vi "Pick&Place_ladder_shih_v11_MPTv2.vi"() -> ()   [LabVIEW 2016]
uses:
  WTF is this.ctl
  Classes/Controllers/I-O/Copy of NI-DAQ Folder/NI-DAQ.lvclass
  D:/INTT/V1/Classes/Controllers/I-O/Copy of I-O Folder/I-O.lvclass
  Classes/Controllers/Dispenser/Copy of Ultimus V2 Folder/Ultimus V2.lvclass
  <vilib>/Analysis/coordinate.llb/2D Cartesian Coordinate Rotation (Scalar).vi
  <vilib>/Utility/file.llb/Read Delimited Spreadsheet (DBL).vi
  <vilib>/Utility/file.llb/Write Delimited Spreadsheet (DBL).vi
  Classes/Controllers/Motion/Copy of Motion Folder/Motion.lvclass
  Classes/Controllers/Camera/Copy of Controller Folder/Controller.lvclass
  <vilib>/Analysis/NI_AALPro.lvlib
  Classes/Controllers/I-O/Copy of I-O Folder/I-O.lvclass
panel:
  out "output array":dbl[](array[numeric])
  in  "Glue hehight":dbl=1.3
  out "file indicator":dbl[][](array[numeric])
  out "?":dbl[](array[numeric]) format="%#_8g"
  in  "offset":dbl[](array[numeric])=[0.0, 0.0, 0.0, 0.0] format="%#_8g"
  out "HDI center positions":dbl[][](array[numeric]) format="%#_8g"
  out "HDI center positions":dbl[][](array[numeric])=[[459.92445114002015, 980.2358762511564, 78.77350133595746, 0.0015214873297426886]] format="%#_8g"
  out "CT sum up":dbl[](array[numeric])
  in  "txt switch":bool
  in  "MPT offset":dbl[][](array[numeric])=[[0.0, 0.0, 0.0, 0.0], [0.0, 0.0, 0.0, 0.0]] format="%#_8g"
  out "CT HPoS":dbl[][](array[numeric]) format="%#_8g"
  out "chip distance by OGP":dbl format="%#_8g"
  out "displacement":dbl[](array[numeric])
  out "gantry position test":dbl[](array[numeric])
  out "gantry target position":dbl[](array[numeric])
  out "chip distance by gantry":dbl format="%#_8g"
  out "after SL":dbl[](array[numeric]) format="%#_8g"
  out "after SR":dbl[](array[numeric]) format="%#_8g"
  out "after NL":dbl[](array[numeric]) format="%#_8g"
  out "S chip":dbl[](array[numeric]) format="%#_8g"
  out "N chip":dbl[](array[numeric]) format="%#_8g"
  in  "?":path=path "C:/Users/PAGANIS/Desktop/shih cheng wei/OGP/test1-2.txt"
  out "bless from OGP !!! Center of  stave":dbl[](array[numeric])
  out "bless from OGP !! measured stave size":dbl[](array[numeric])
  in  "Bless from OGP":bool
  out "FROM Detail !!! Center of module on stave":dbl[](array[numeric])
  out "FROM Detail !! measured stave size":dbl[](array[numeric])
  in  "Align Stave in detail":bool
  in  "Uttimus presssure":i64=10
  out "Status":bool
  out "measured HDI top-left position":dbl[][](array[numeric])
  in  "HDI vacuum channel":i32=18
  in  "vacuum":bool=TRUE
  in  "HDI vacuum":bool
  out "measured stave size":dbl[](array[numeric])
  out "Stave mark":dbl[][](array[numeric])
  out "Center of module on stave":dbl[](array[numeric])
  out "Measured HDI size":dbl[][](array[numeric])
  out "MPT positions on stave":T1[][](array[typedef])
  in  "Default Stave dimension":dbl[](array[numeric])=[34.0, 472.0, -0.335295, -0.000320234]
  in  "Default Stave upper left mark":dbl[](array[numeric])=[584.376, 675.576, 70.9882, 0.000840064]
  out "Needle parking position":dbl[](array[numeric])
  in  "Uppler / Lower Stave":bool=TRUE
  out "Gantry current position":dbl[](array[numeric])
  in  "READ Position":bool
  in  "Needle Height Compenstation\n(glue gap)":dbl=0.33
  in  "Needle Alignment":bool
  in  "Parking position":dbl[](array[numeric])=[625.0, 625.0, 0.0, 0.01]
  in  "GOTO":bool
  in  "Default Pickup Tool Position":dbl[][](array[numeric])=[[152.226, 682.729, 36.8129, -0.0151898], [700.0, 800.0, 20.0, 0.01]]
  in  "deposit glue module":i32=1
  in  "Default HDI alignment \nmark position":dbl[](array[numeric])=[448.322, 976.582, 74.9872, 0.000191129]
  in  "Default HDI size":dbl[](array[numeric])=[24.2437, 231.446, -0.099339, 0.000191129]
  out "# of tasks excuted":i32
  out "PickupTool \nCenterPosition":dbl[](array[numeric]) format="%#_8g"
  in  "Inititalize":bool
  in  "Pick and place":bool
  in  "Deposit Glue":bool
  in  "Measure Pickup Tools":bool
  in  "Align Stave":bool
  out "default module position on stave":dbl[][](array[numeric])
  in  "Stop":bool
  in  "Measure HDI":bool
  # "Ladder Assembly"
  # "To switch the north/south\ntxt file \nswitch \noffset\nmodule pick up tool\nmodule direction"
  # "upper : north \nlower : south"
  # "Sensor 0.32 -> 200 micron glue thickness\nChips 0.37-> 140 micron glue thickness"
  # "Upper\nmodule"
  # "Lower\nmodule"
  # "ACTIONS"
  # "theta had *-1"
  # "Pick up tool and needle"
  # "Module infomation"
  # "Pick and Place"
  # "after assembly"
  # "CT"
  # "+"
  # "+"
  # "="
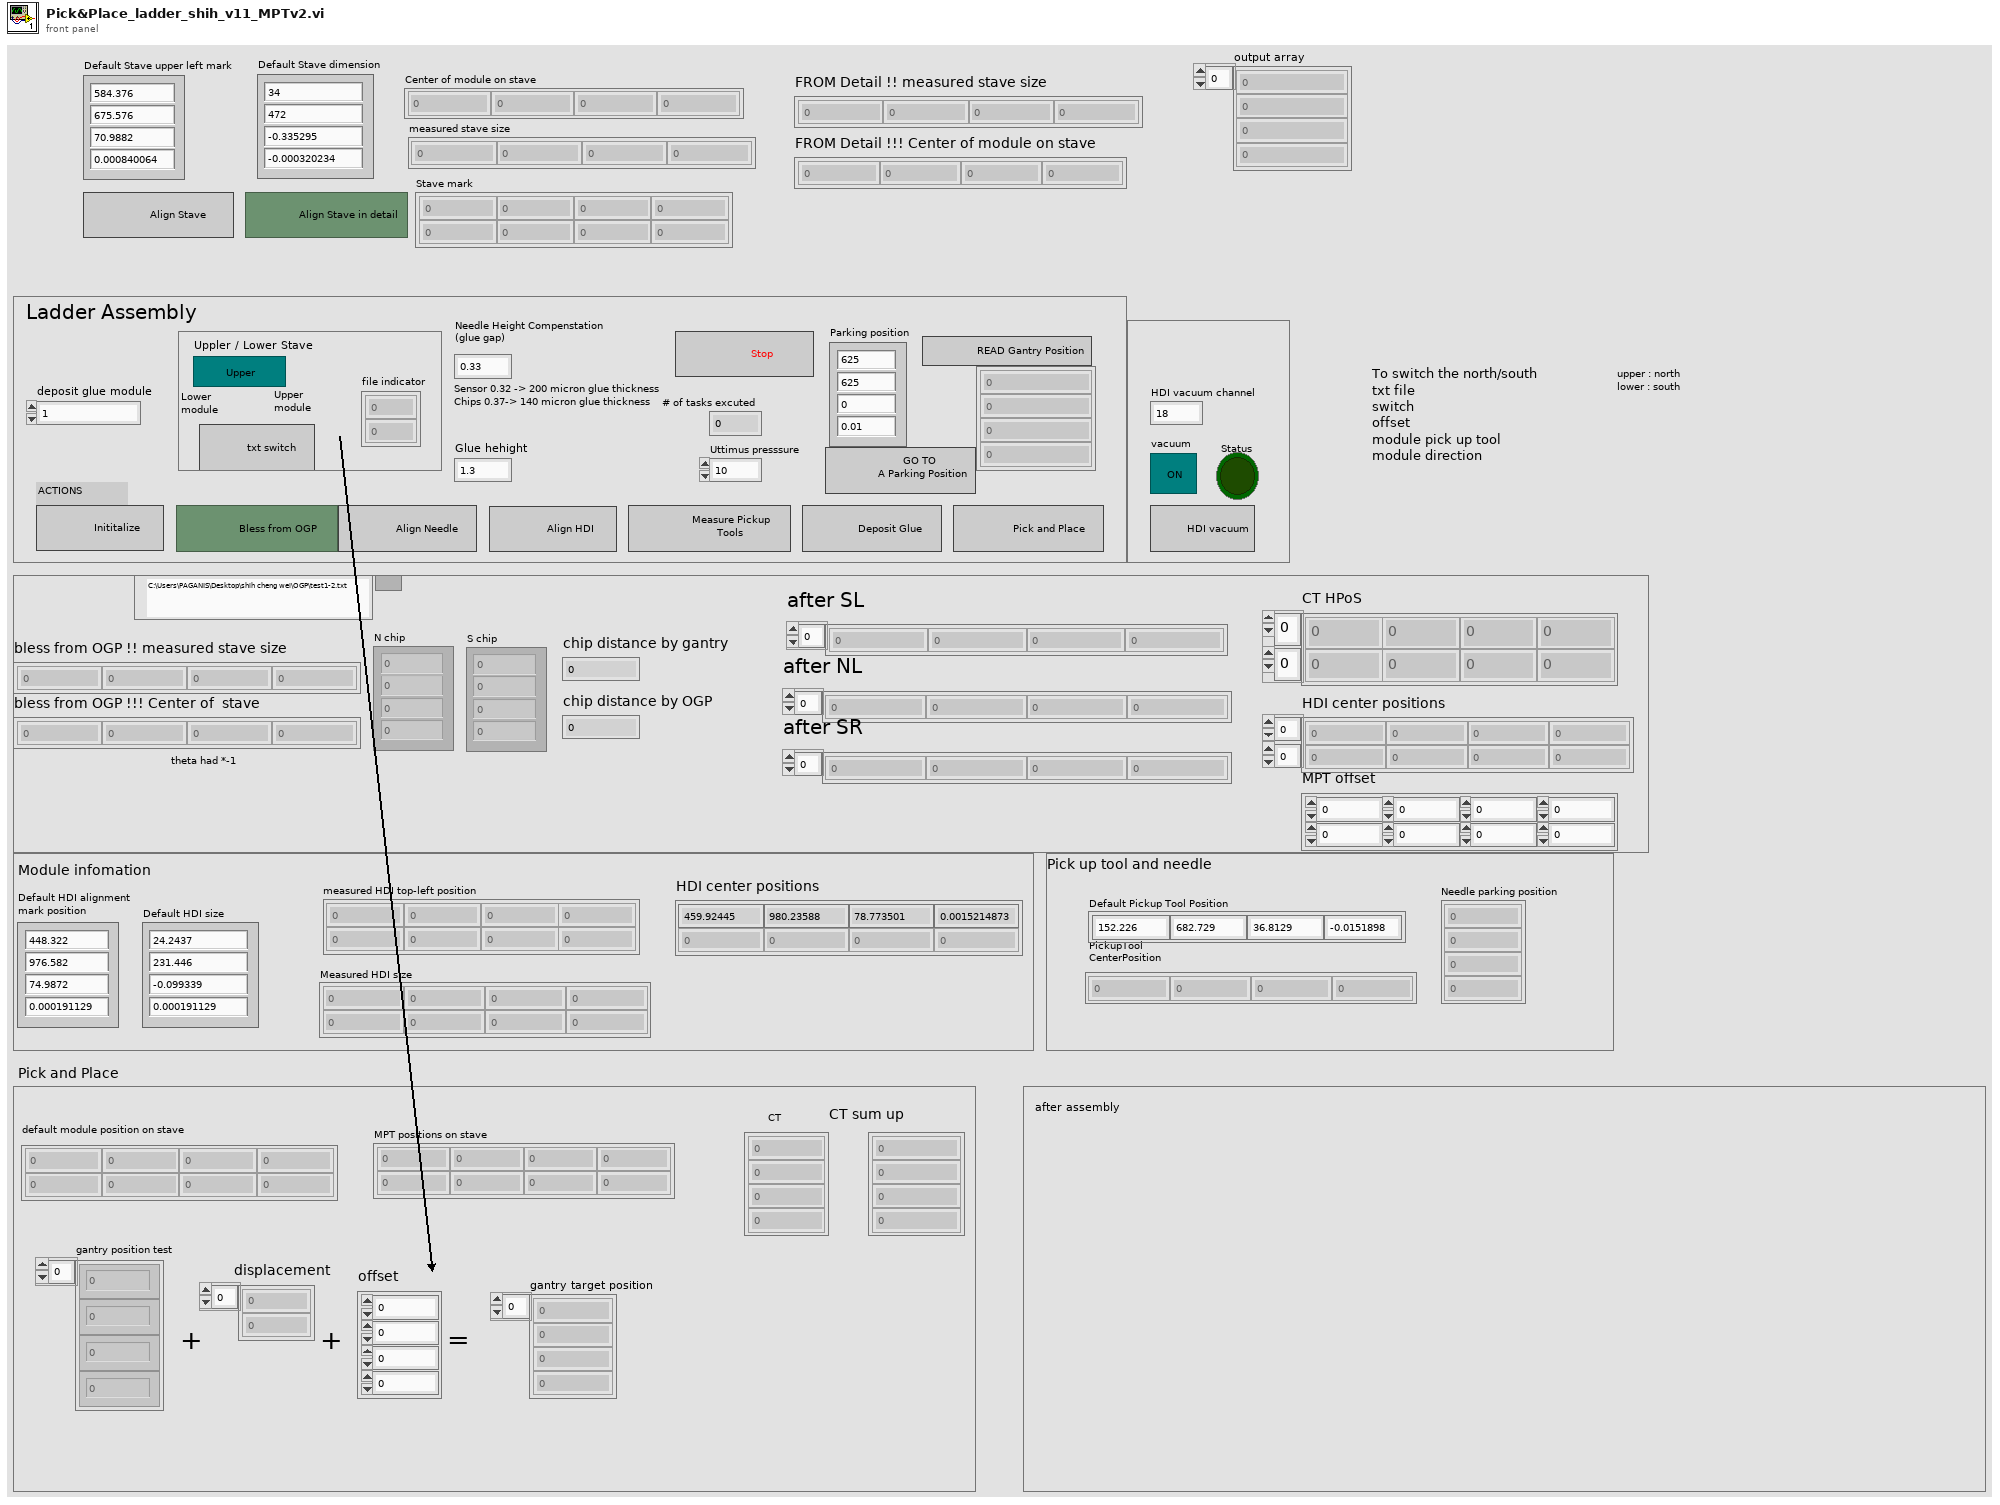
[diagram p1: front panel]
types:
  T1 = typedef "WTF is this.ctl" = dbl
  T2 = typedef "Controller.lvclass/Controllers.ctl" = cluster{"Copy of Motion.lvclass":refnum<class "Motion.lvclass">, "Copy of I-O.lvclass":refnum<class "I-O.lvclass">, "Copy of Dispenser.lvclass":refnum<class "Dispenser.lvclass">}
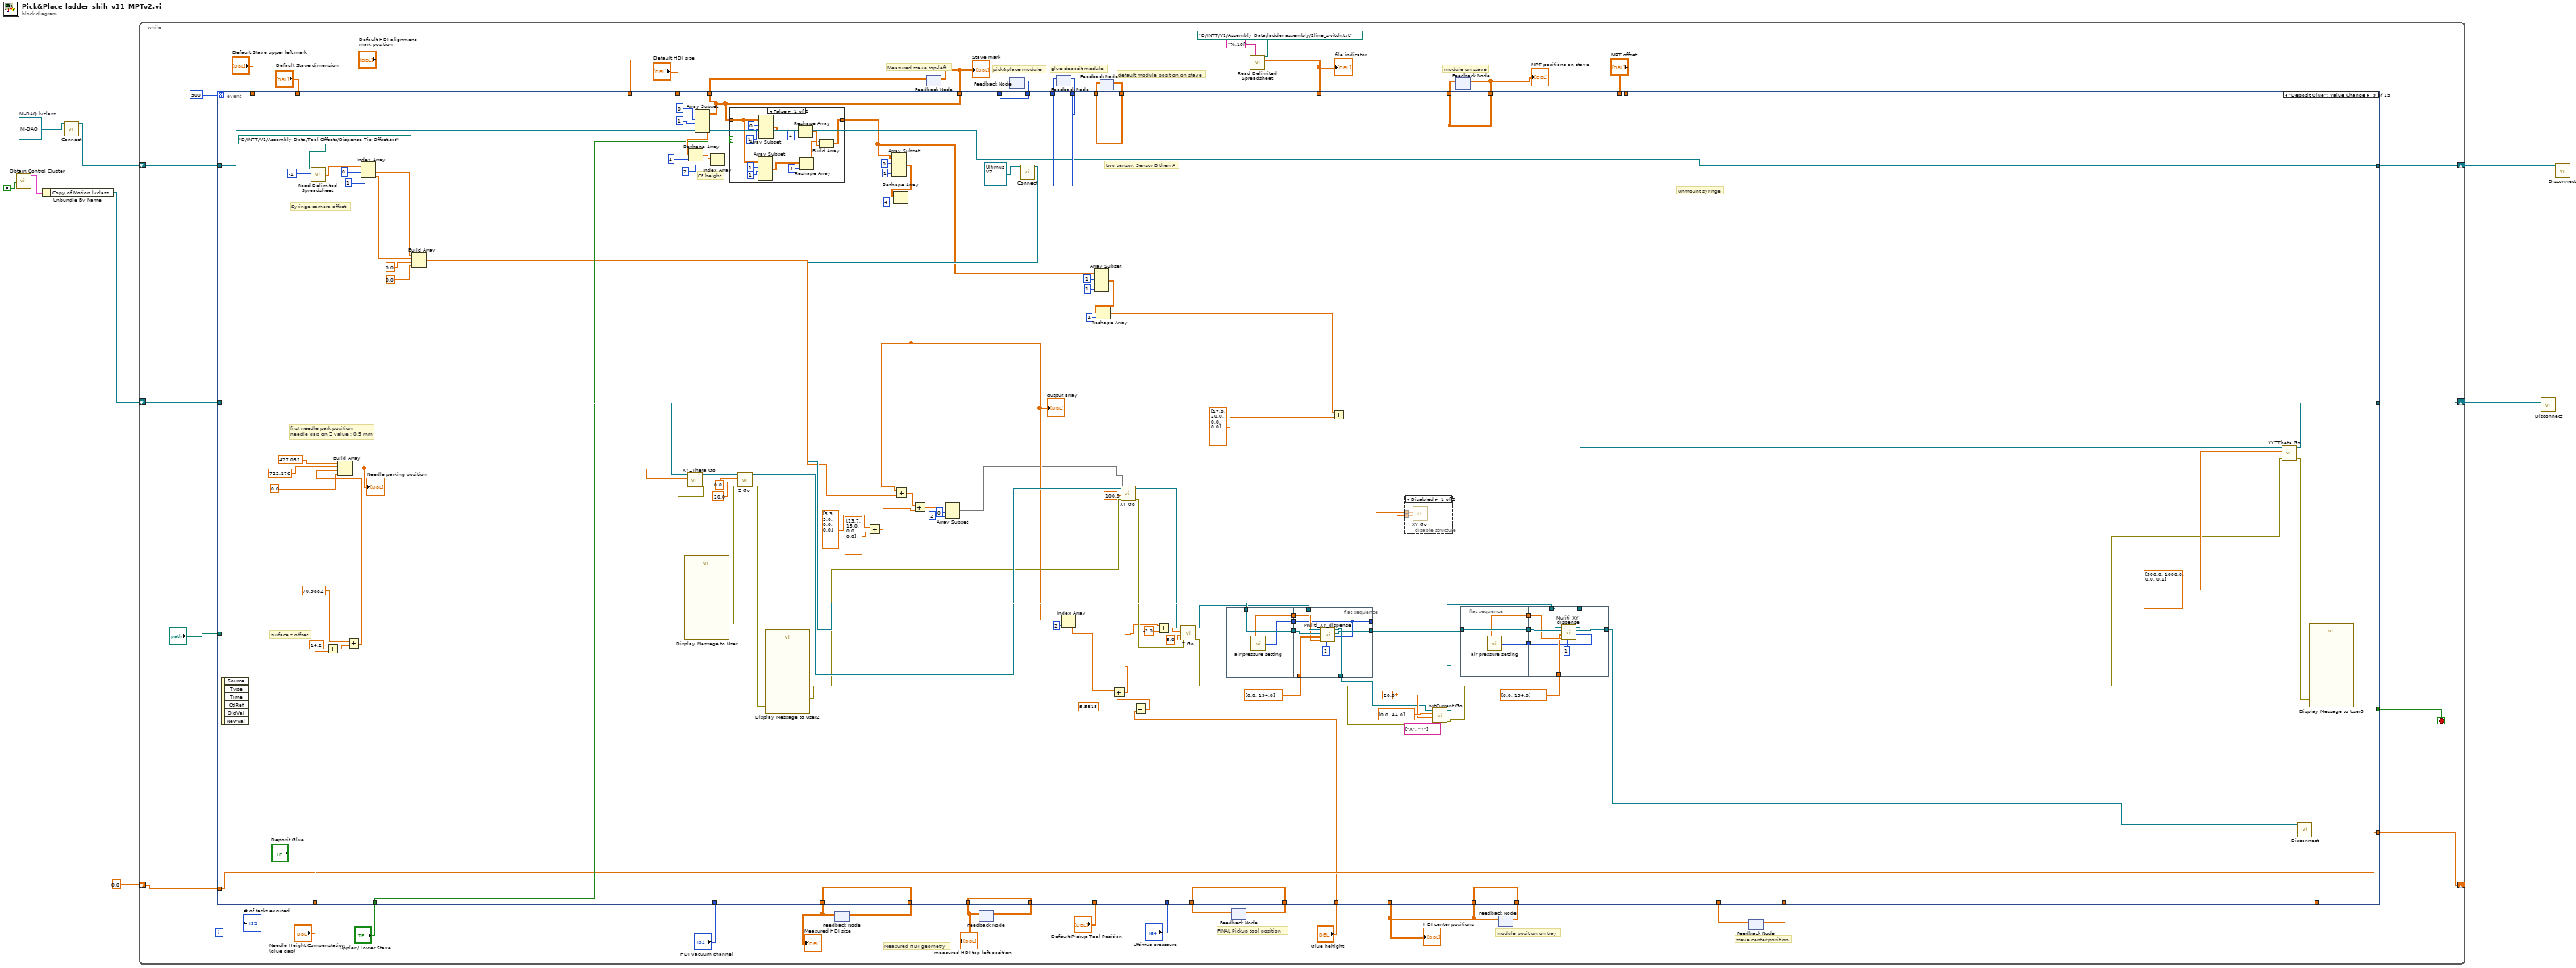
[diagram p0: block diagram]
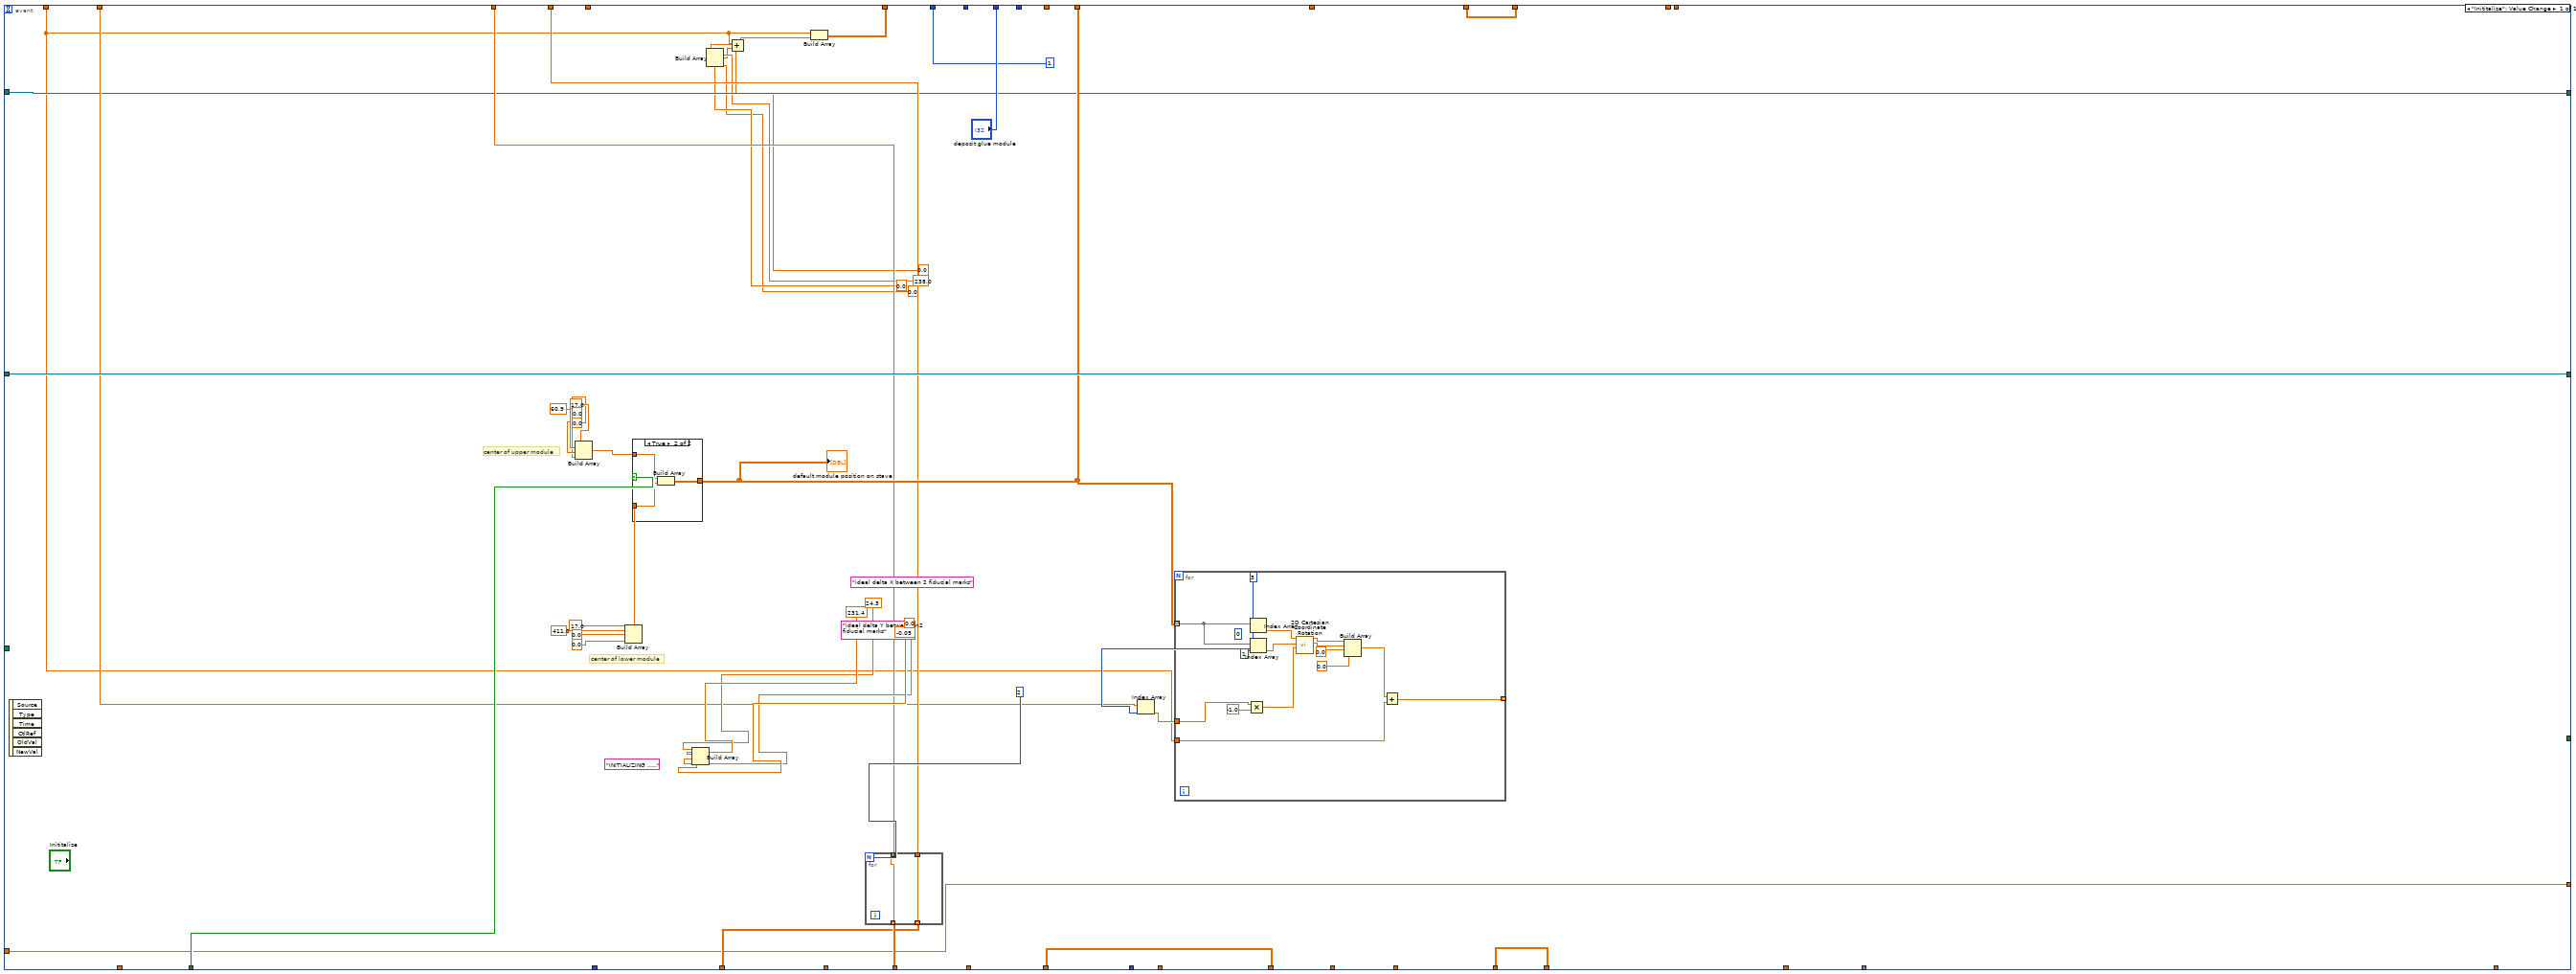
[diagram p2: hidden frame]
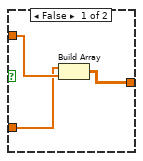
[diagram p3: hidden frame]
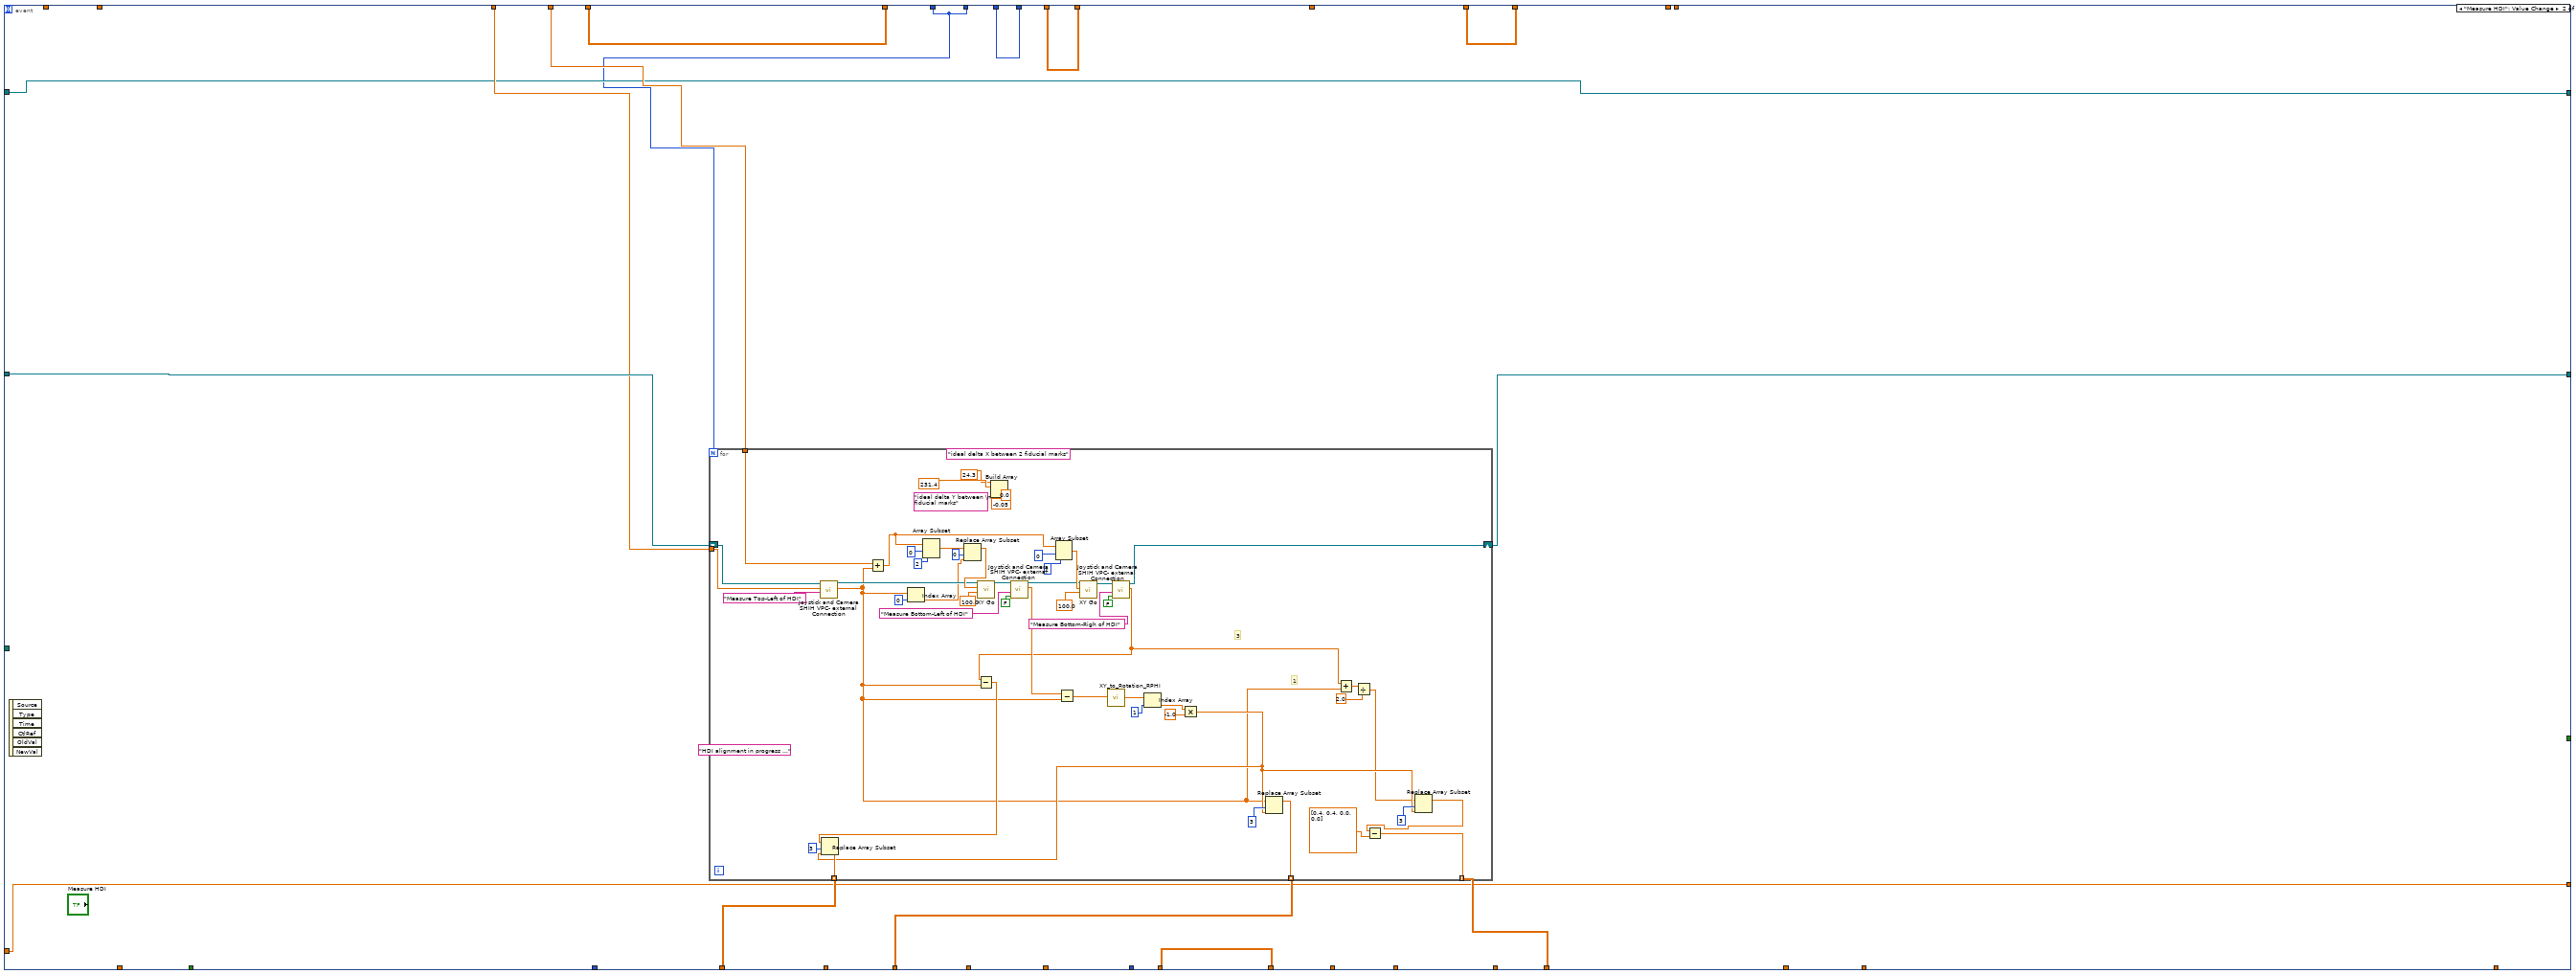
[diagram p4: hidden frame]
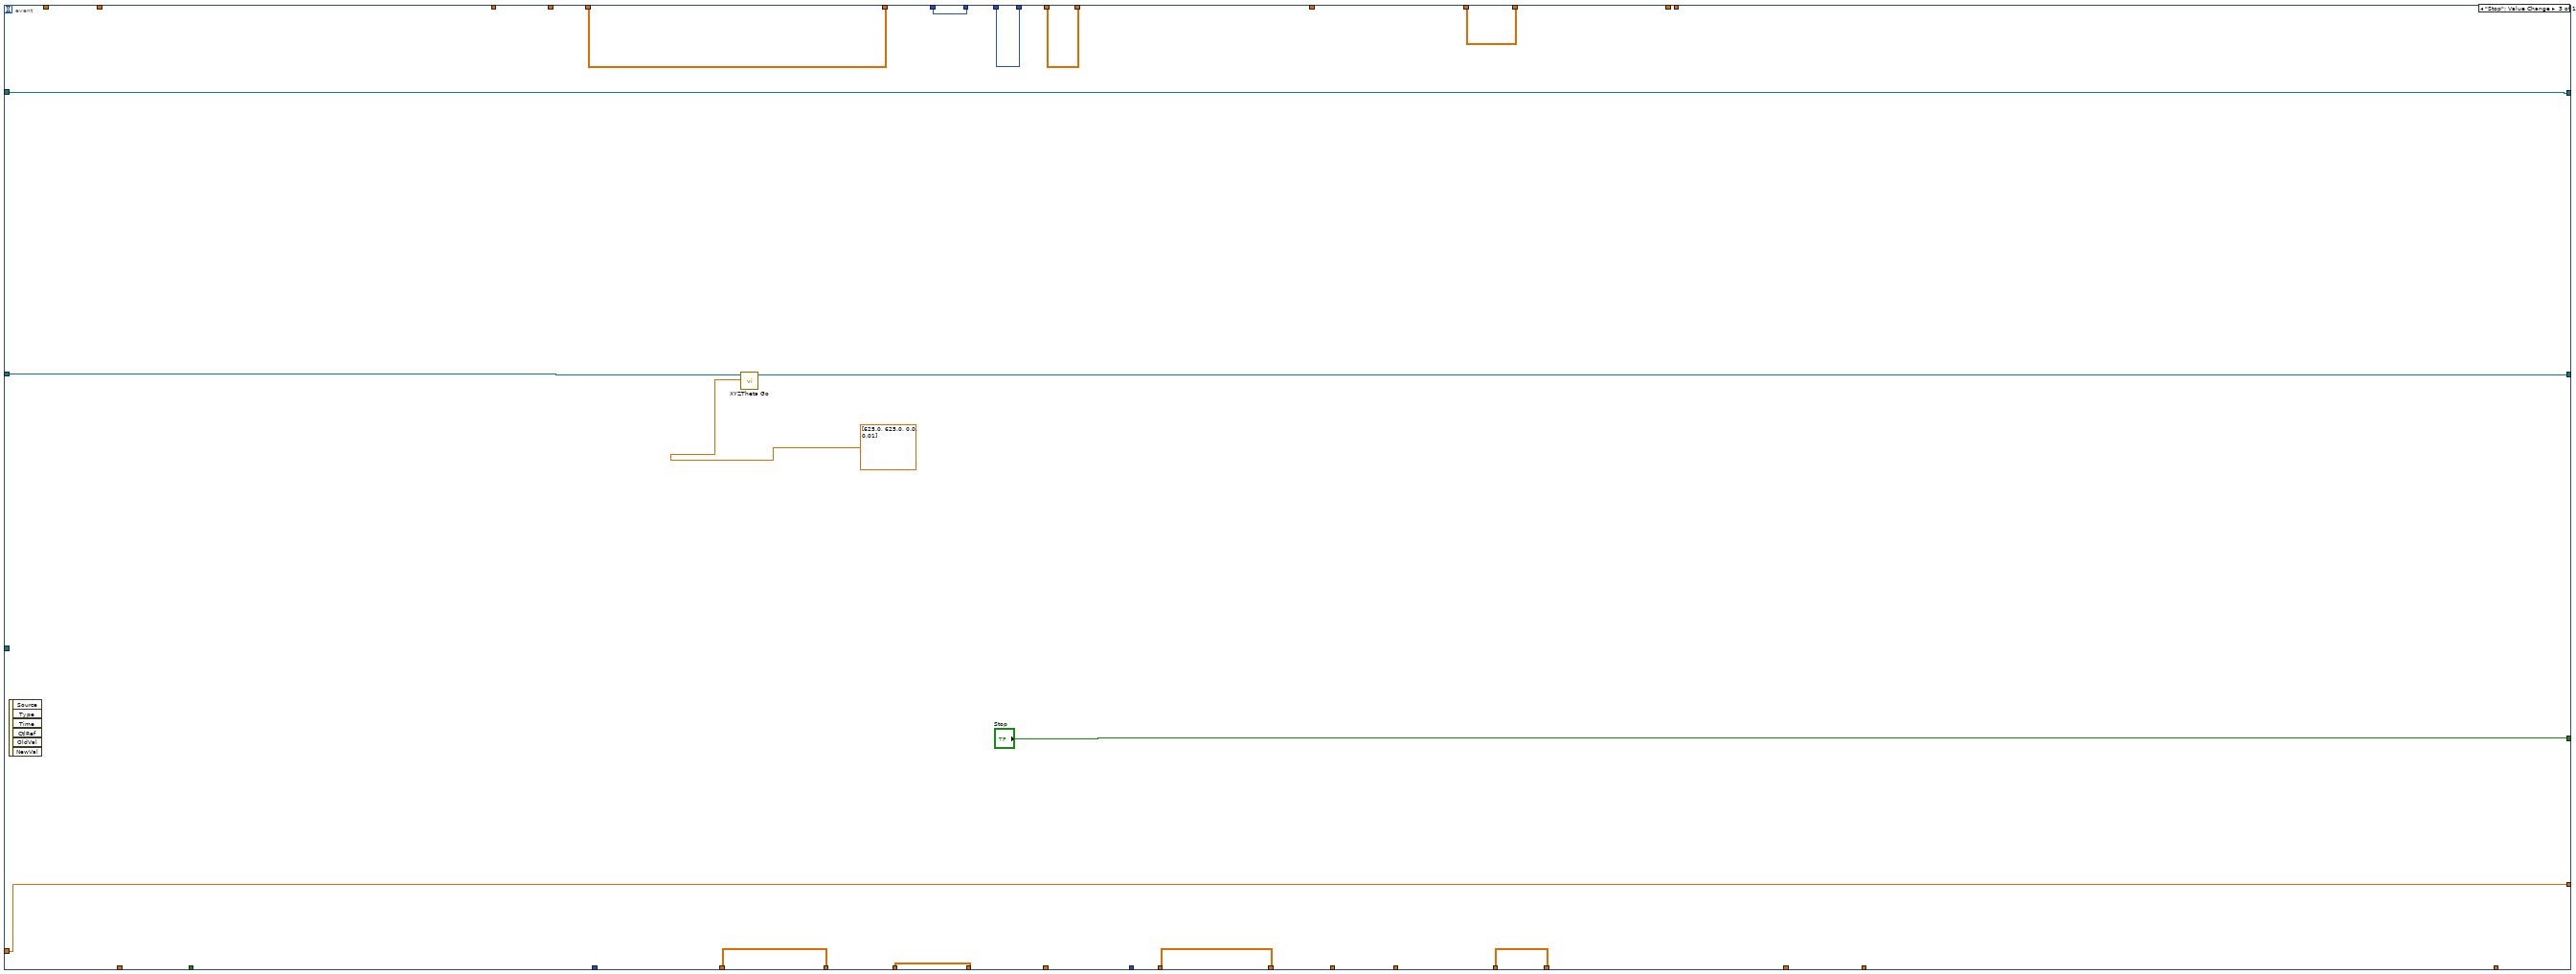
[diagram p5: hidden frame]
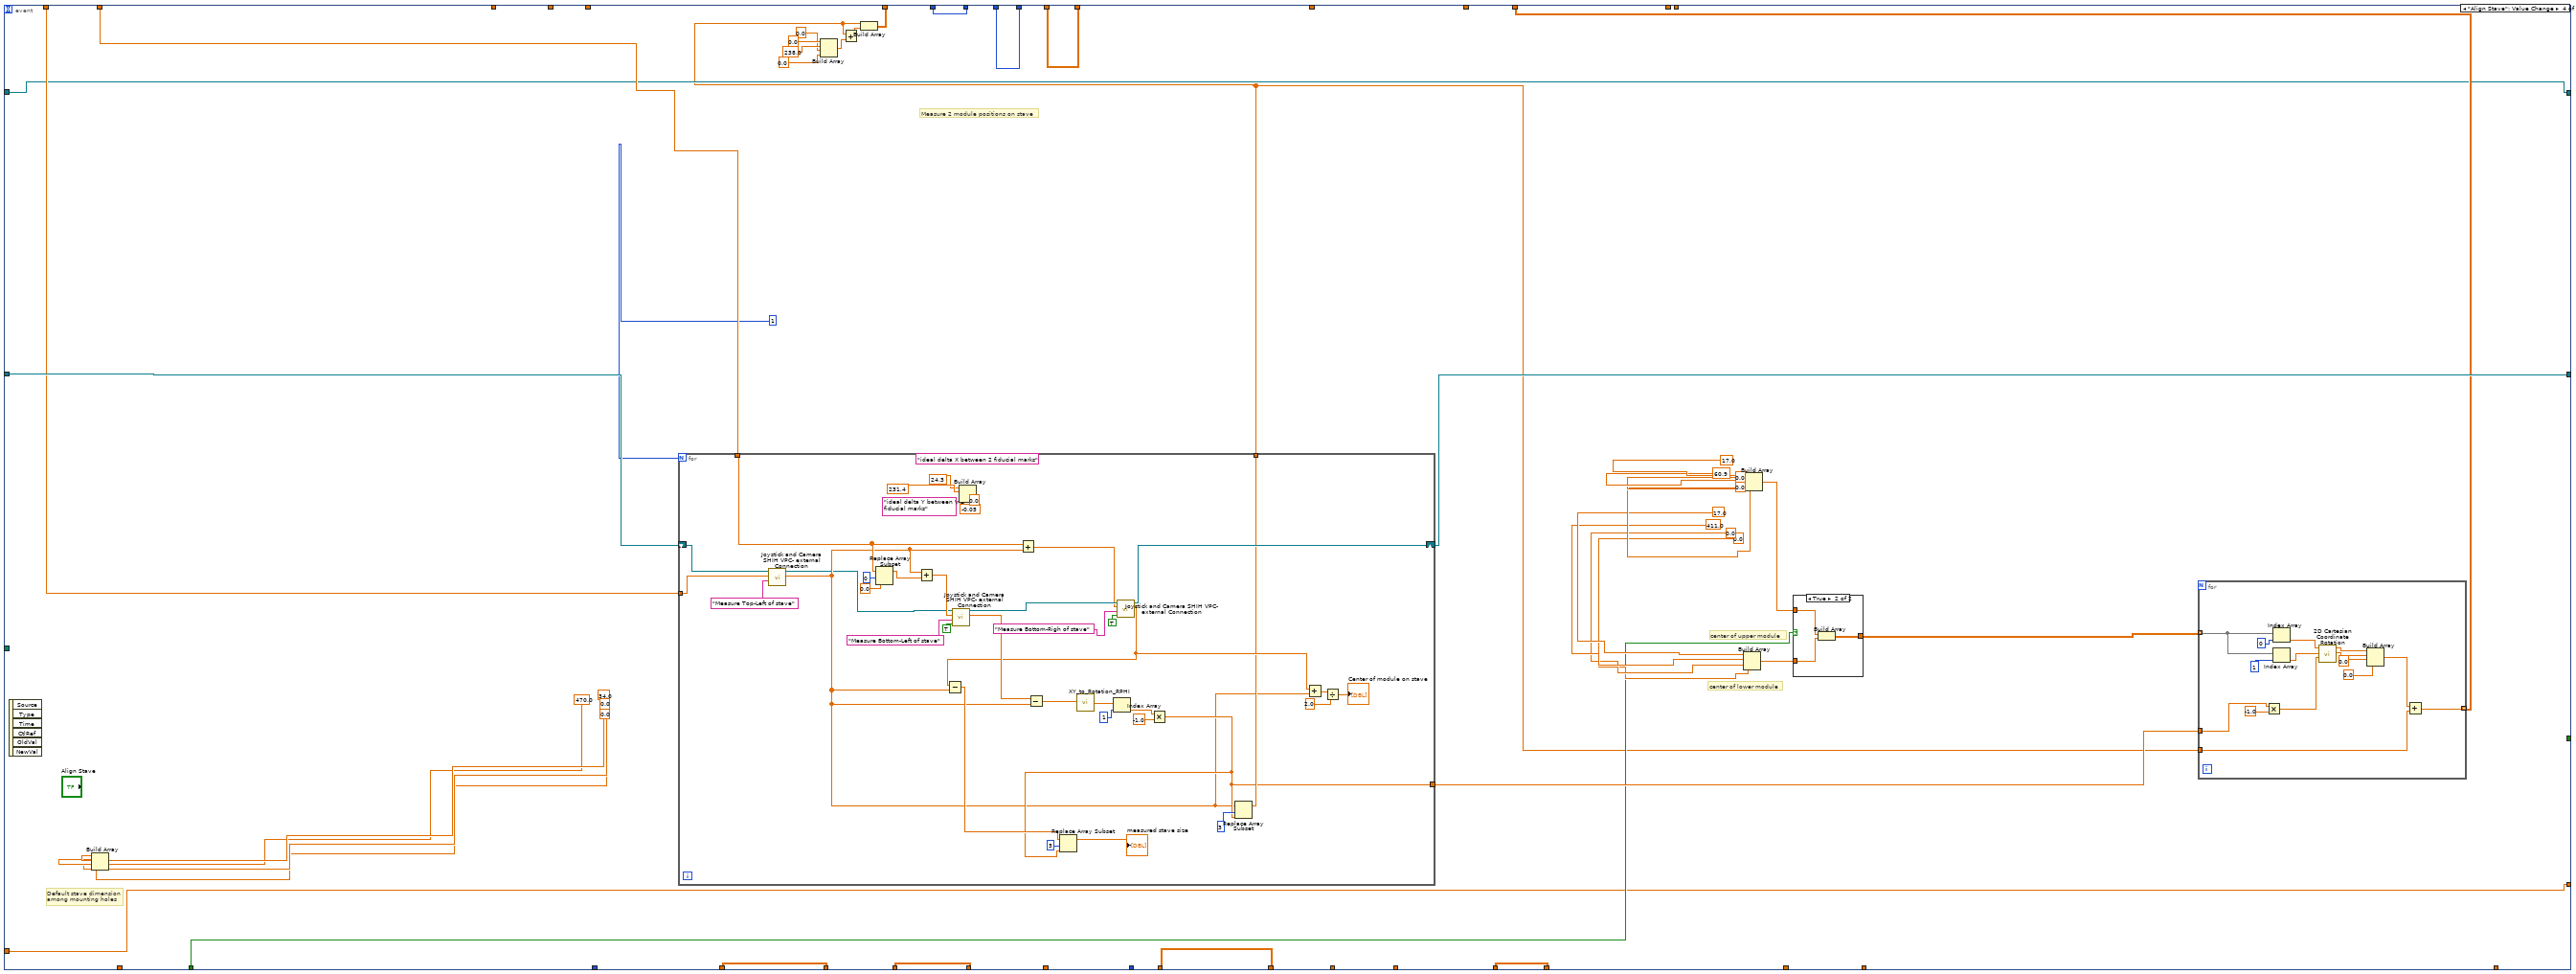
[diagram p6: hidden frame]
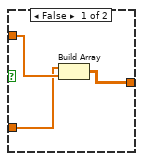
[diagram p7: hidden frame]
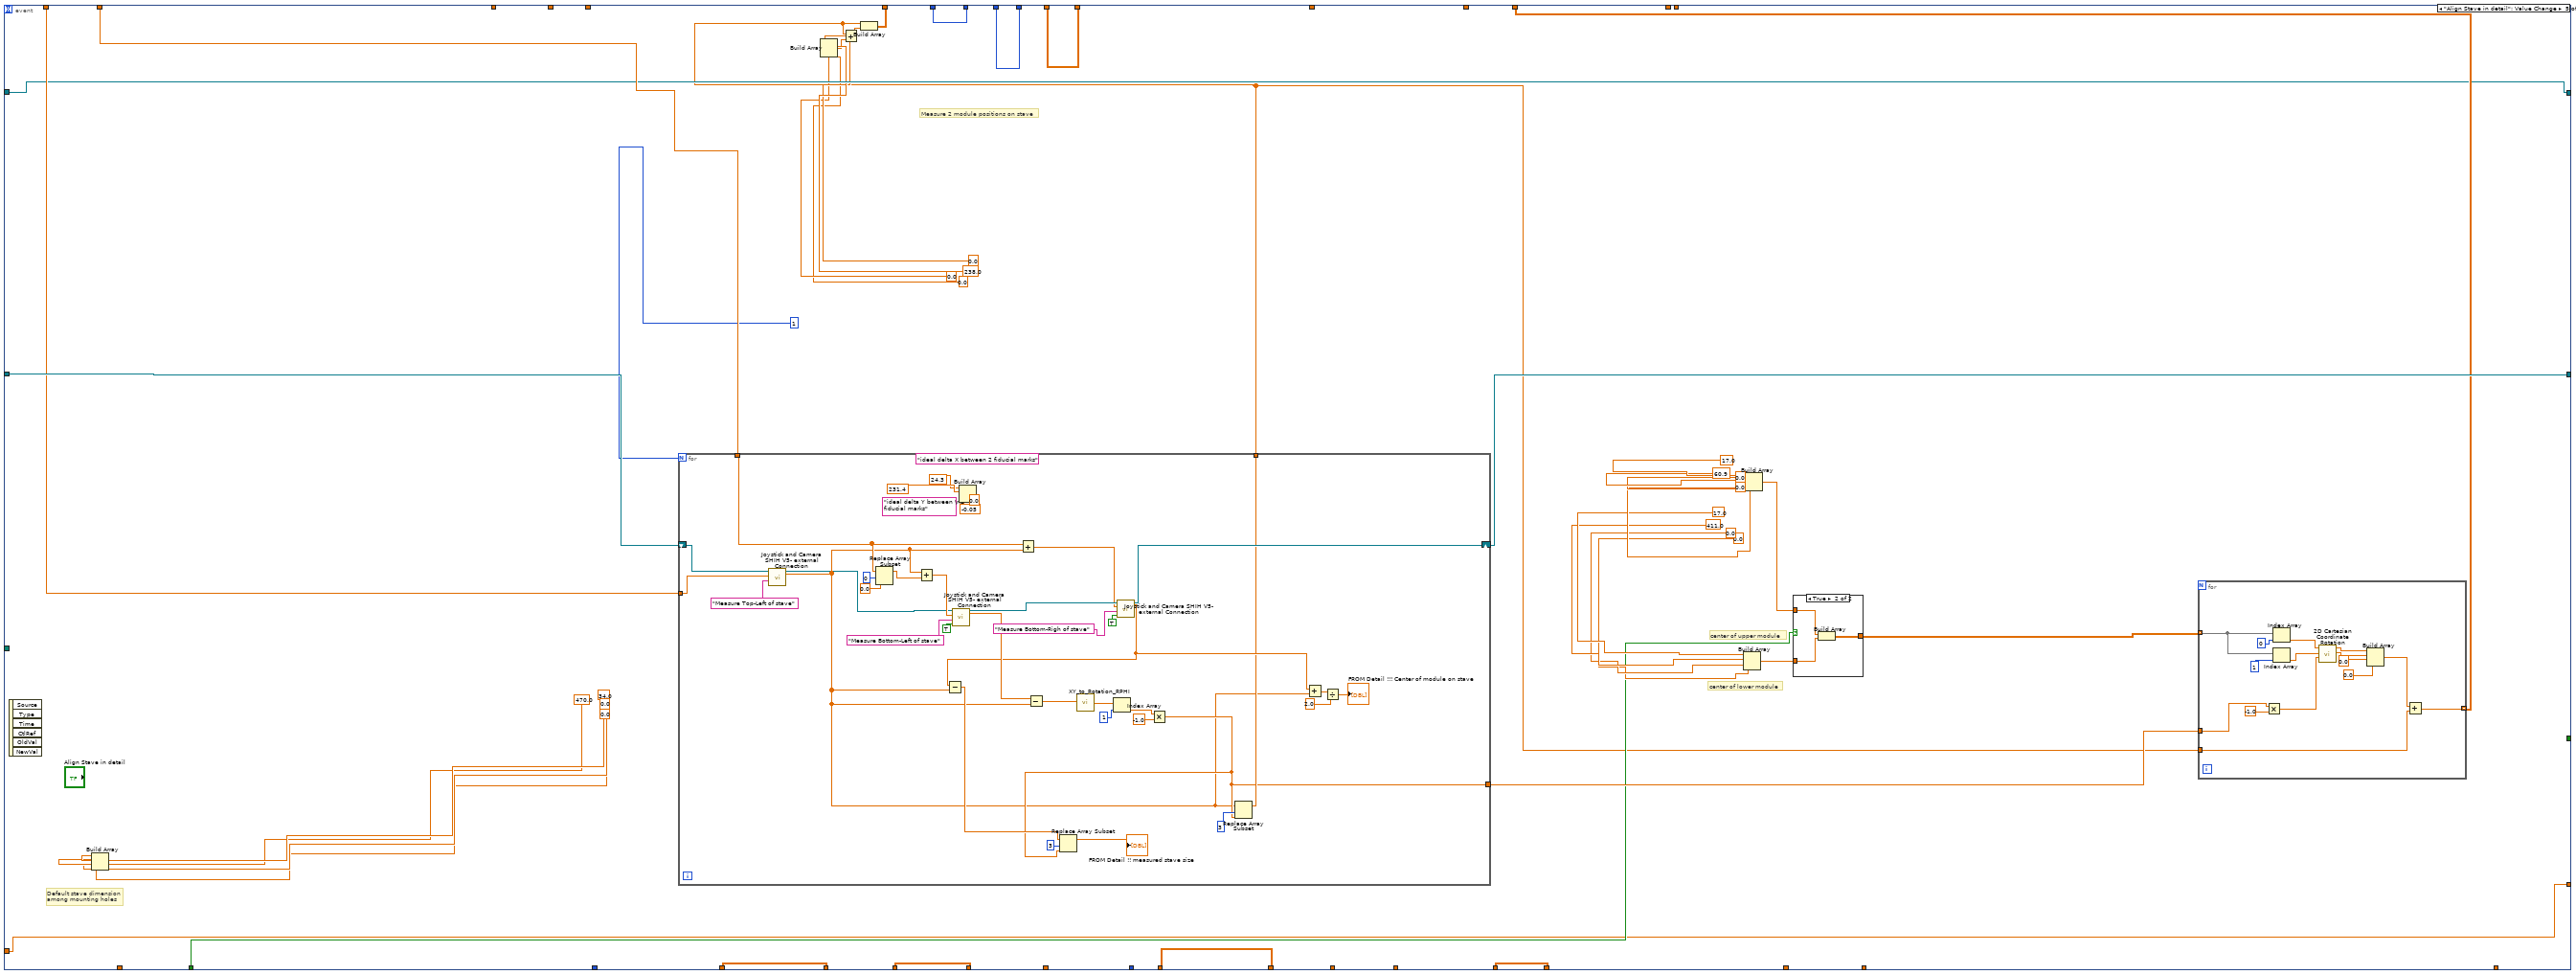
[diagram p8: hidden frame]
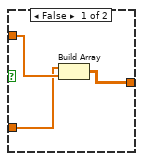
[diagram p9: hidden frame]
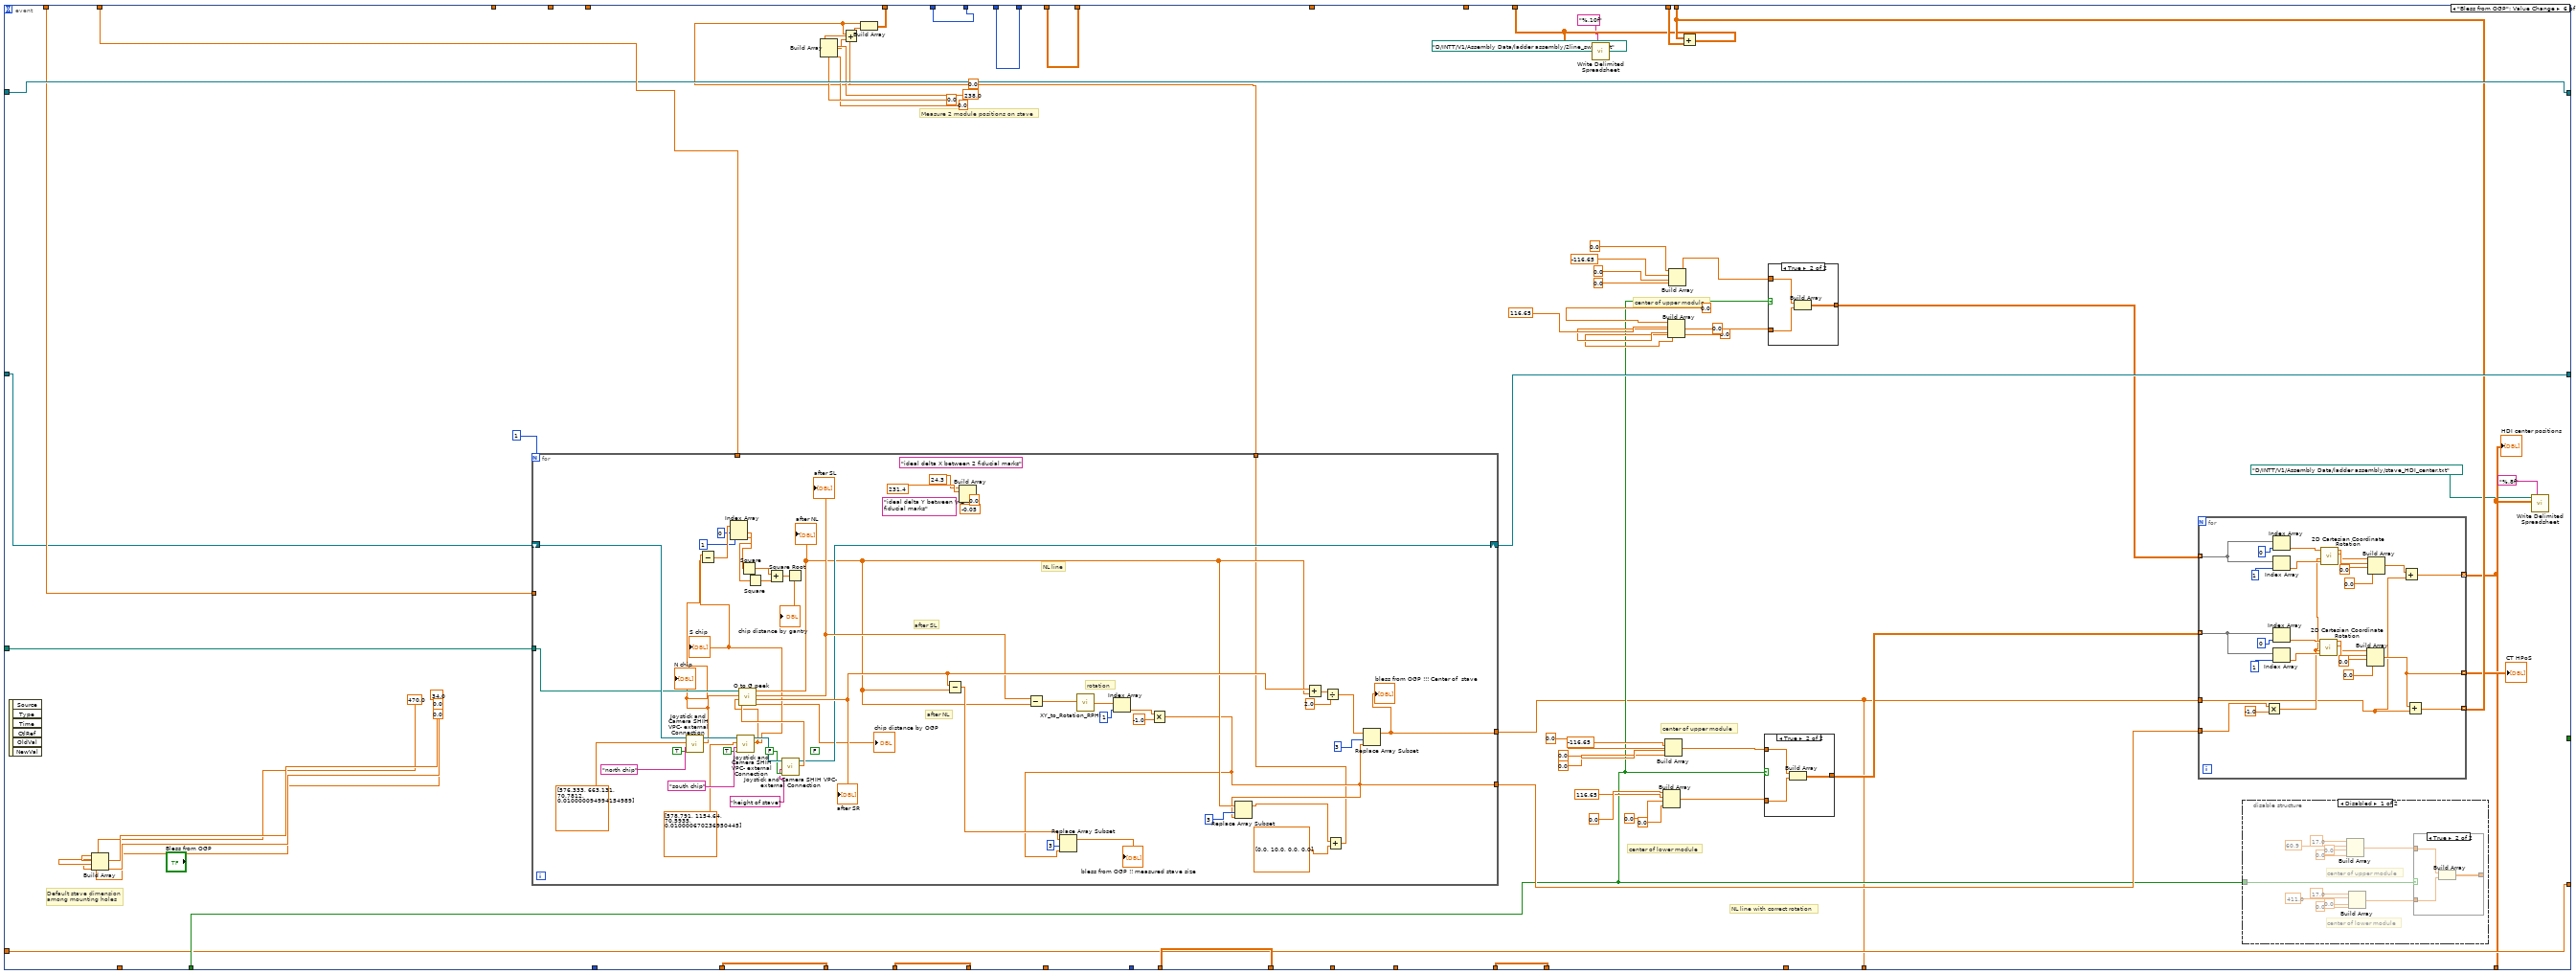
[diagram p10: hidden frame]
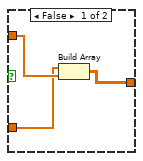
[diagram p11: hidden frame]
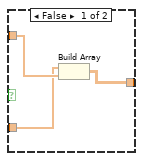
[diagram p12: hidden frame]
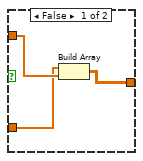
[diagram p14: hidden frame]
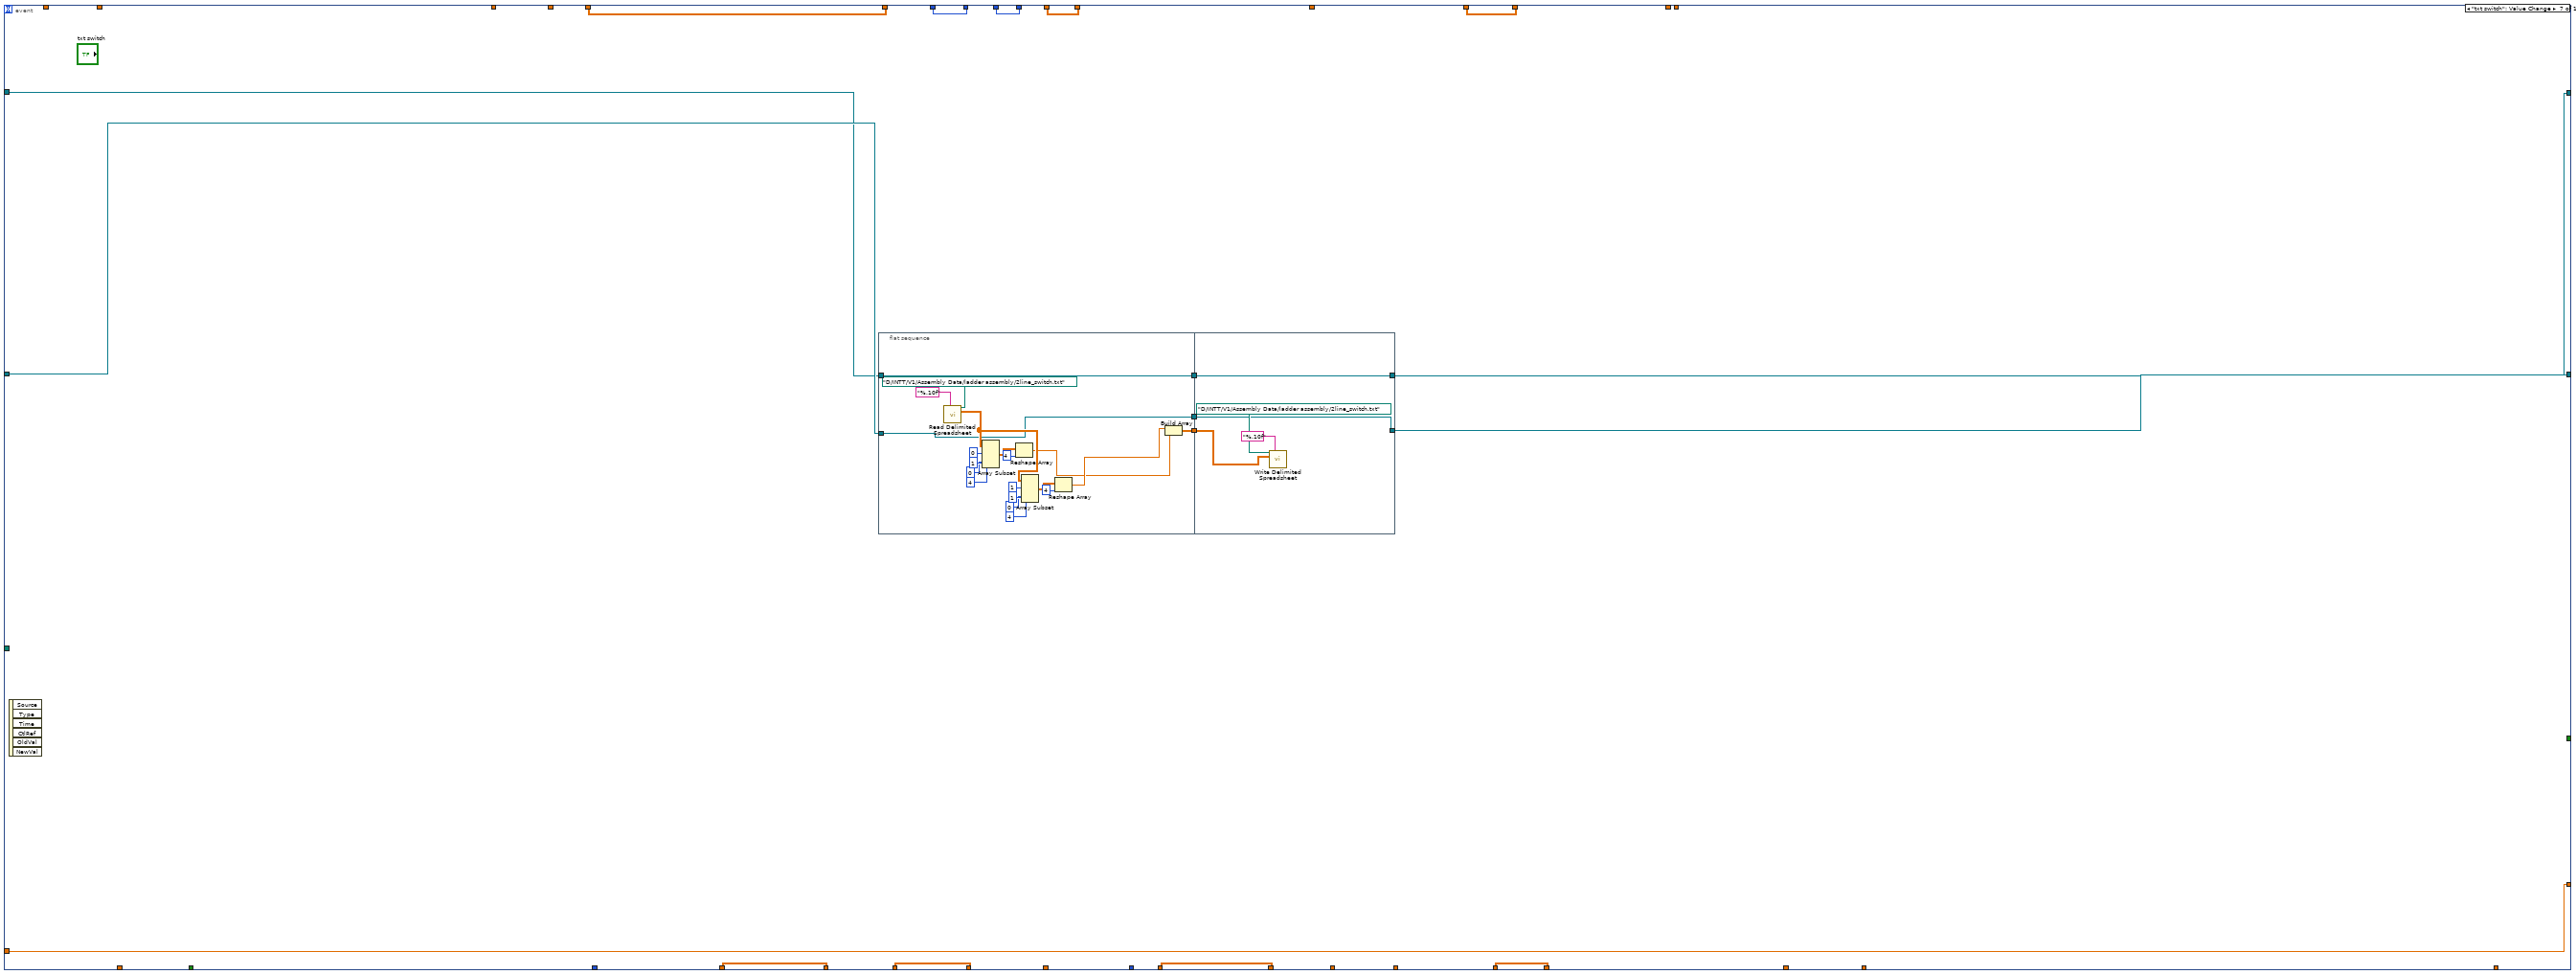
[diagram p15: hidden frame]
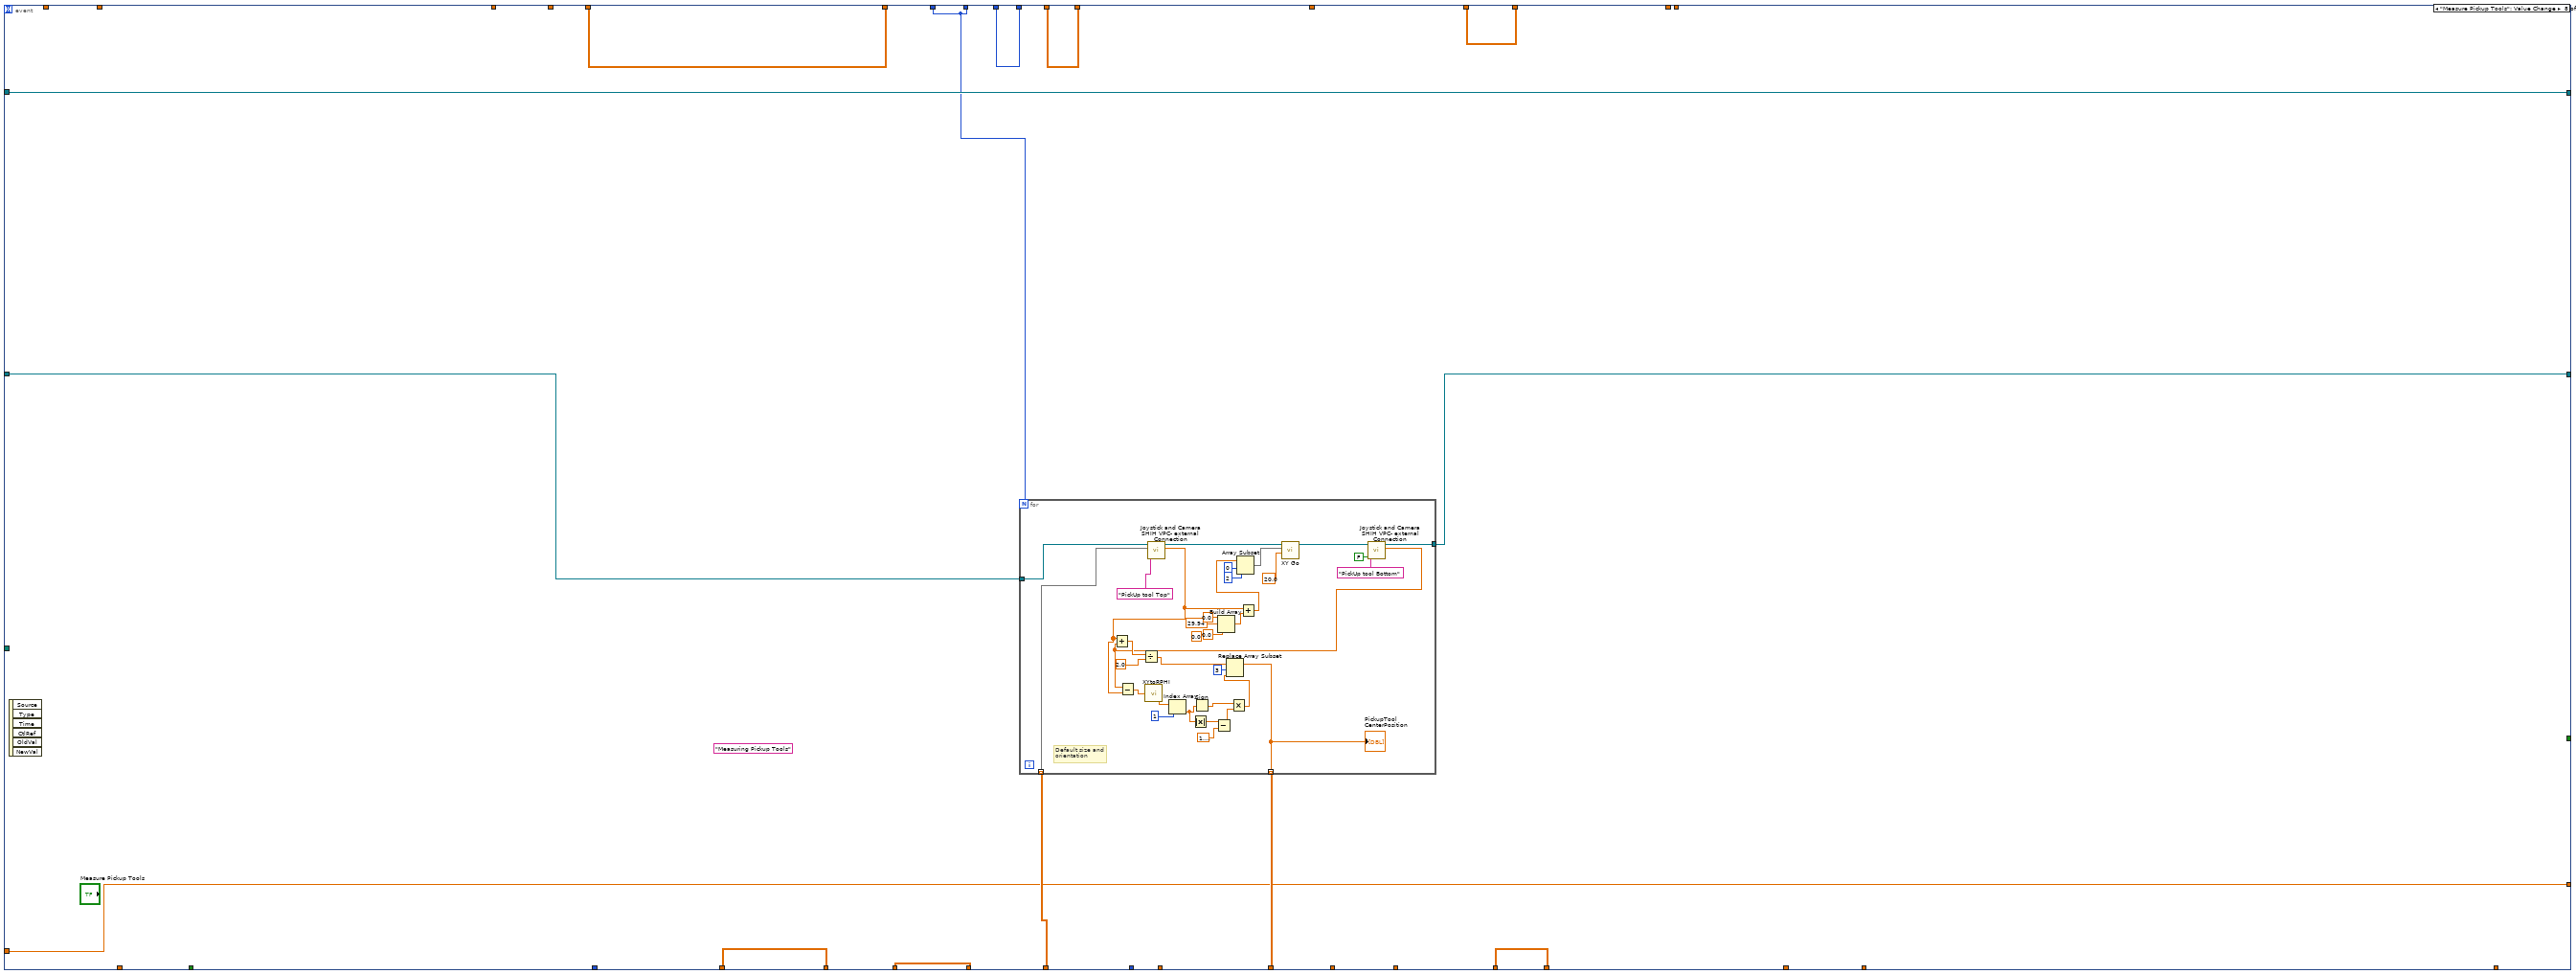
[diagram p16: hidden frame]
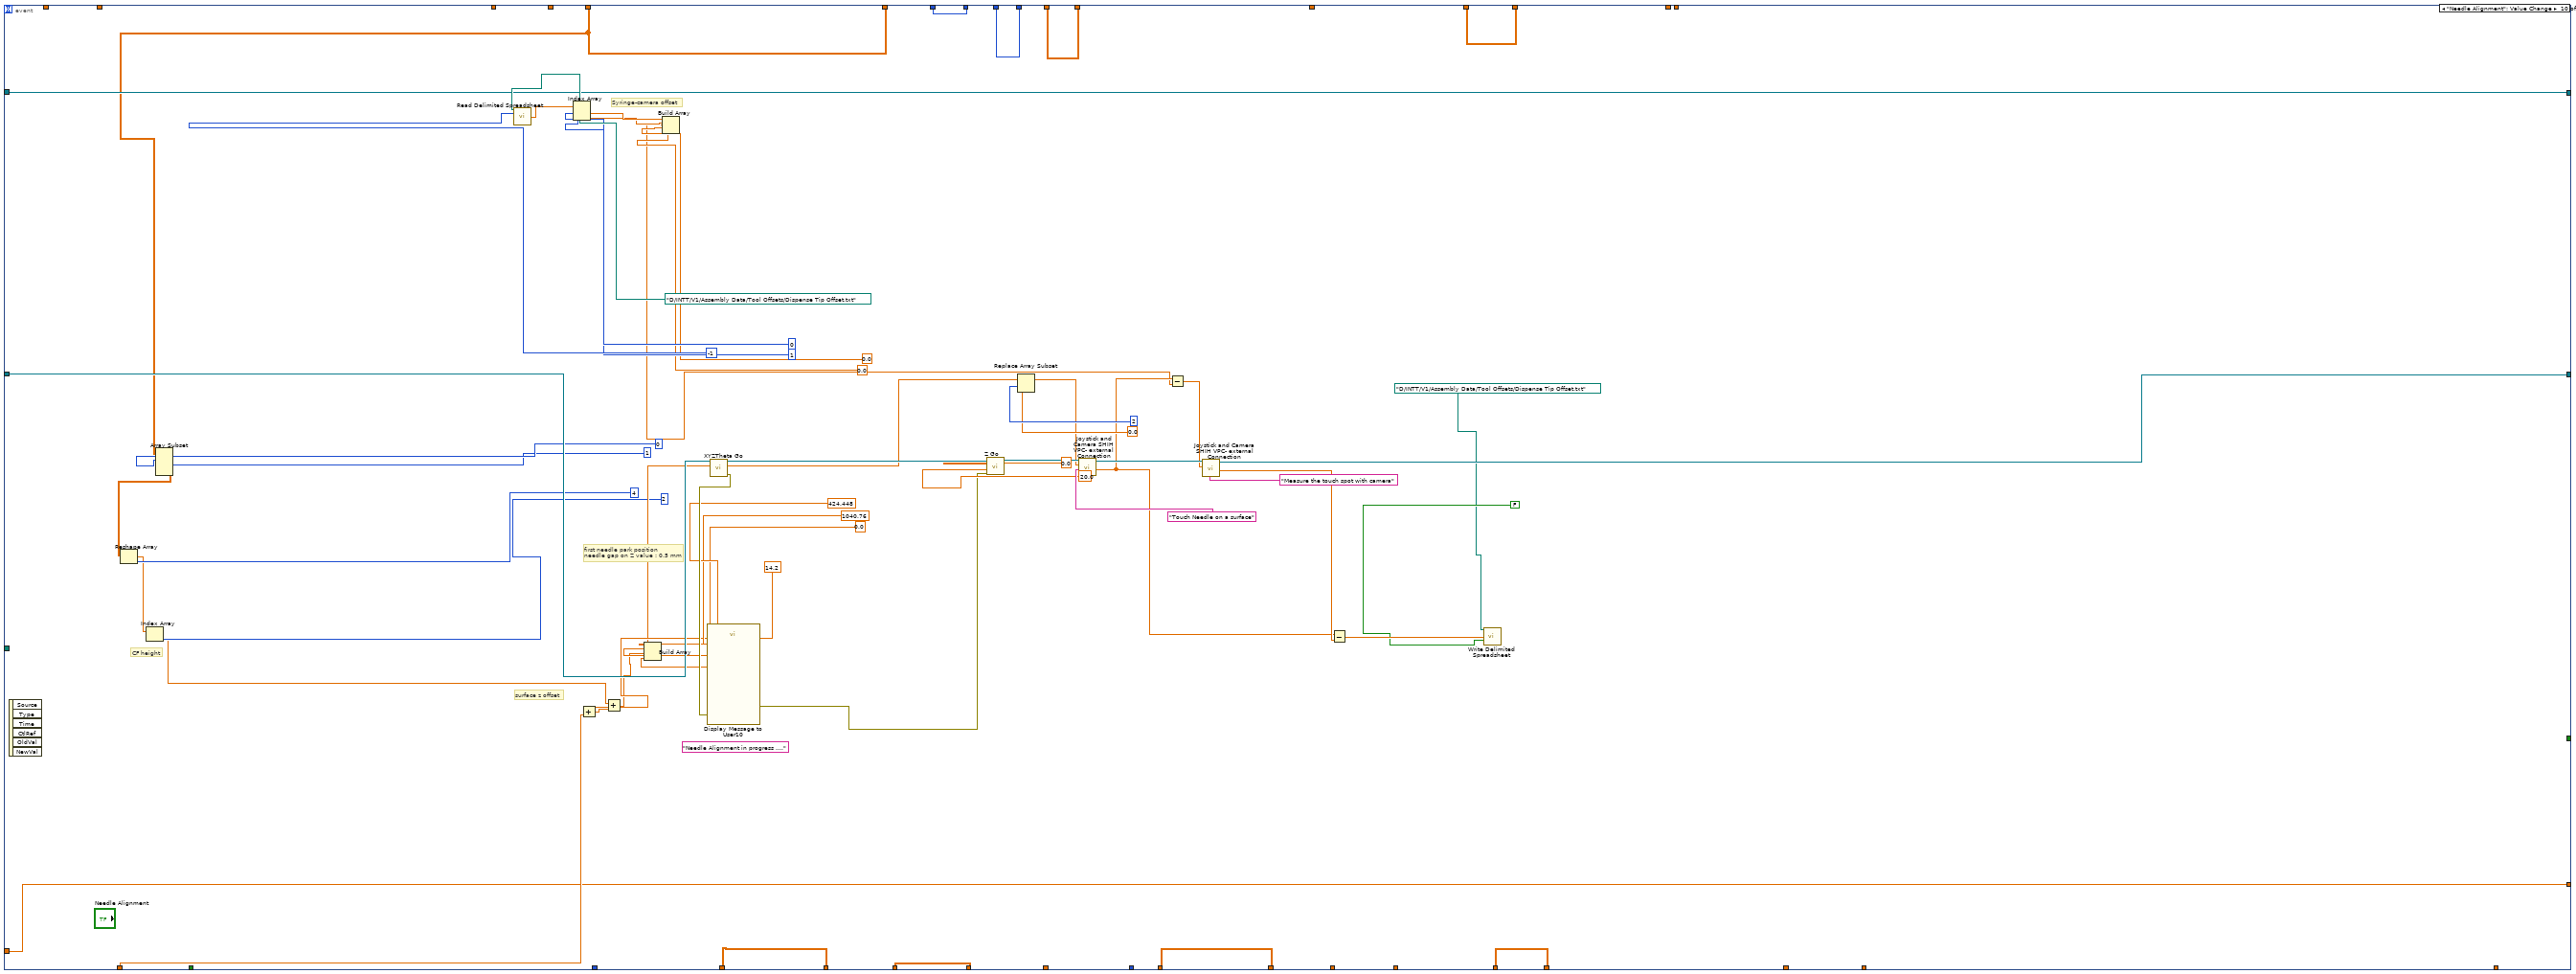
[diagram p19: hidden frame]
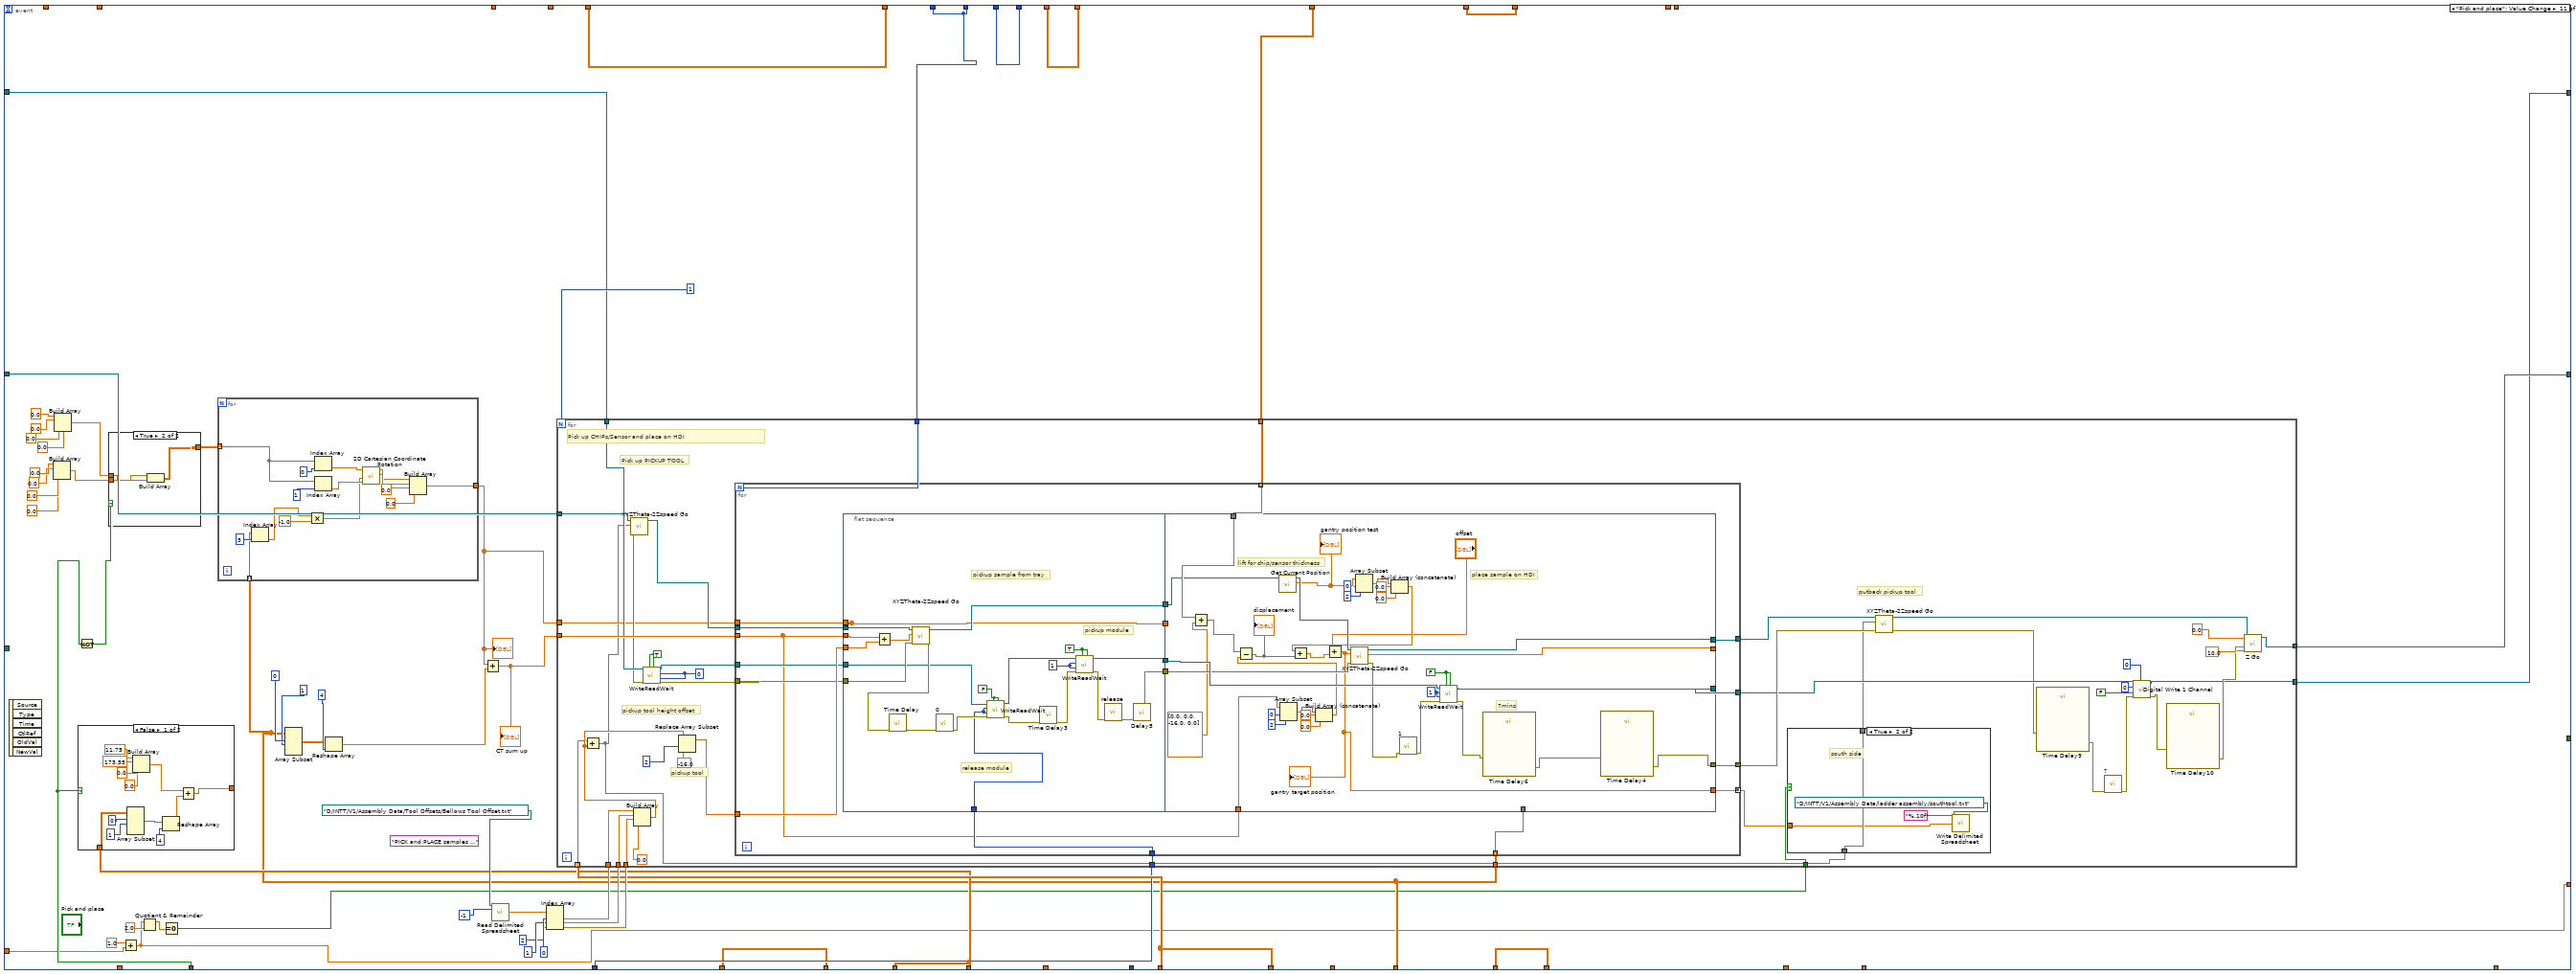
[diagram p20: hidden frame]
diagram:
  w4 = refnum<class "NI-DAQ.lvclass"> refnum  # NI-DAQ.lvclass
  n1 = call "Obtain Control Cluster.vi"("I/O"=FALSE) -> ("Control Out"=w8:T2)  [unwired: 10 in]
  n2 = Unbundle By Name(w8) -> ("Copy of Motion.lvclass"=w6:refnum<class "Motion.lvclass">)
  n3 = call-dynamic "Connect.vi"("NI-DAQ in"=w4) -> ("NI-DAQ out"=w3:refnum<class "NI-DAQ.lvclass">)  [unwired: 9 in, 1 out]
  n4 = while {
    shift-right: [w45] -> w5
    shift-left: w6 -> [w52]
    shift-right: [w25] -> w2
    shift-left: w3 -> [w29]
    shift-right: [w12] -> _
    shift-left: 0.0 -> [w13]
    i -> [w44]
    stop <- w51 stop-if-true
    # "stave center position"
    # "pick&place module"
    # "default module position on stave"
    # "FINAL Pickup tool position"
    # "glue deposit module"
    # "Measured HDI geometry"
    # "module position on tray"
    # "Measured stave top-left"
    # "module on stave"
    n5 = feedback #1() -> (w49:dbl[][])  [unwired: 1 in]
    n6 = feedback #2() -> (w50:dbl[][])  [unwired: 1 in]
    n7 = feedback #3() -> (w26:dbl[][])  [unwired: 1 in]
    n8 = feedback #4() -> (w15:i32)  [unwired: 1 in]
    n9 = feedback #5() -> (w43:i32)  [unwired: 1 in]
    n10 = feedback #6() -> (w38:dbl[][])  [unwired: 1 in]
    n11 = feedback #7() -> (w46:dbl[][])  [unwired: 1 in]
    n12 = call-poly <vilib>:"Read Delimited Spreadsheet.vi"("file path (dialog if empty)"=path "D:/INTT/V1/Assembly Data/ladder assembly/2line_switch.txt" ("file path (dialog if empty) 3"), "format (%.3f)"="%.10f") -> ("all rows"=w17:dbl[][])  [unwired: 8 in, 5 out]
    "file indicator" <- w17
    n13 = feedback #8() -> (w33:dbl[][])  [unwired: 1 in]
    n14 = feedback #9() -> (w14:dbl[][])  [unwired: 1 in]
    "HDI center positions" <- w14
    n15 = feedback #10() -> (w10:dbl[])  [unwired: 1 in]
    n16 = event shown="[8] \"Deposit Glue\": Value Change" {
      selector: _ -> [_ _ _ _ _ _ _ _ _ _ _ _ _ _ _]
      dyn-events: _ -> [_ _ _ _ _ _ _ _ _ _ _ _ _ _ _]
      timeout: 500 -> [_ _ _ _ _ _ _ _ _ _ _ _ _ _ _]
      tunnel: w52 -> [w88 w129 w195 w227 w325 w427 w565 w614 w736 w826 w897 w1075 w1095 w1099 w1122]
      tunnel: [_ _ "Stop" _ _ _ _ _ _ _ _ _ _ _ _] -> w51
      tunnel: [w56 w123 w190 w198 w296 w430 w570 w609 w706 w792 w878 w1081 w1091 w1107 w1121] -> w30
      tunnel: w50 -> [_ w123 w190 _ _ _ w570 w609 w706 w792 w878 w1081 w1091 w1107 w1121]
      tunnel: [w66 w121 w189 w223 w321 w442 w574 w608 w725 w829 w880 w1078 w1090 w1101 w1119] -> w31
      tunnel: w49 -> [_ _ w189 w223 w321 w442 w574 w608 w725 w829 w880 w1078 w1090 w1101 w1119]
      tunnel: w43 -> [_ w116 w192 w228 w326 w445 w569 w605 w728 w831 w874 w1080 w1092 w1105 w1113]
      tunnel: [w71 w120 w187 w230 w328 w447 w571 w607 w727 w827 w865 w1076 w1088 w1103 w1116] -> w48
      tunnel: w14 -> [w71 _ w187 w230 w328 w447 w571 w607 w727 w827 w865 w1076 w1088 w1103 w1116]
      tunnel: [w86 w124 w188 w235 w333 w452 w572 w613 w726 w828 w886 w1077 w1089 w1102 w1117] -> w47
      tunnel: w46 -> [_ w124 w188 w235 w333 w452 w572 _ w726 w828 w886 w1077 w1089 w1102 w1117]
      tunnel: [w88 w128 w193 w224 w322 w443 w563 w612 w729 w818 w887 w1073 w1094 w1099 w1122] -> w45
      tunnel: ["deposit glue module" w116 w192 w228 w326 w445 w569 w605 w728 w831 w874 w1080 w1092 w1105 w1113] -> w42
      tunnel: "Default HDI alignment \nmark position" -> [w69 w127 _ _ _ _ _ _ _ _ _ _ _ _ _]
      tunnel: "Default HDI size" -> [w68 w126 _ _ _ _ _ _ _ _ _ _ _ _ _]
      tunnel: [w75 w125 w191 w229 w327 w446 w568 w610 w724 w830 w885 w1079 w1093 w1106 w1120] -> w39
      tunnel: w38 -> [_ w125 w191 w229 w327 w446 w568 w610 w724 w830 w885 w1079 w1093 w1106 w1120]
      tunnel: "Default Pickup Tool Position" -> [w86 _ _ _ _ _ _ w611 _ _ _ _ _ _ _]
      tunnel: "Uppler / Lower Stave" -> [w72 _ _ w208 w306 w398 _ _ w712 _ w854 _ _ _ _]
      tunnel: "Default Stave upper left mark" -> [w57 _ _ w226 w324 w429 _ _ _ _ _ _ _ _ _]
      tunnel: "Default Stave dimension" -> [w65 _ _ w225 w323 w444 _ _ _ _ _ _ _ _ _]
      tunnel: [w54 w122 w185 w207 w305 w412 w567 w606 w723 w809 w876 w1071 w1085 w1104 w1115] -> w32
      tunnel: w33 -> [w54 w122 w185 _ _ _ w567 w606 w723 w809 w876 w1071 w1085 w1104 w1115]
      tunnel: w29 -> [w64 w118 w183 w206 w304 w438 w562 w603 w718 w807 w883 w1070 w1084 w1111 w1125]
      tunnel: [w64 w118 w183 w206 w304 w438 w560 w603 w718 w807 w882 w1070 w1084 w1098 w1123] -> w25
      tunnel: "HDI vacuum channel" -> [_ _ _ _ _ _ _ _ _ _ w881 _ _ w1108 w1124]
      tunnel: [w67 w119 w184 w222 w320 w441 w573 w604 w719 w808 w879 w1072 w1086 w1100 w1118] -> w27
      tunnel: w26 -> [_ _ w184 w222 w320 w441 w573 w604 w719 w808 w879 w1072 w1086 w1100 w1118]
      tunnel: "Needle Height Compenstation\n(glue gap)" -> [_ _ _ _ _ _ _ _ w713 w800 _ _ _ _ _]
      tunnel: "Uttimus presssure" -> [_ _ _ _ _ _ _ _ _ _ _ _ _ _ _]
      tunnel: "?" -> [_ _ _ _ _ w428 _ _ _ _ _ _ _ _ _]
      tunnel: [_ _ _ _ _ w426 _ _ _ _ _ _ _ _ _] -> _
      tunnel: "MPT offset" -> [_ _ _ _ _ w413 _ _ _ _ _ _ _ _ _]
      tunnel: w17 -> [_ _ _ _ _ _ _ _ _ _ w877 _ _ _ _]
      tunnel: [1 ("pick &place module") w117 w182 w197 w295 w409 w566 w602 w705 w790 w875 w1069 w1083 w1097 w1114] -> w16
      tunnel: w15 -> [_ w117 w182 w197 w295 w409 w566 w602 w705 w790 w875 w1069 w1083 w1097 w1114]
      tunnel: w14 -> [_ _ _ _ _ _ _ _ _ _ w855 _ _ _ _]
      tunnel: [_ _ _ _ _ w395 _ _ _ _ _ _ _ _ _] -> _
      tunnel: w13 -> [w53 w115 w181 w196 w294 w396 w559 w601 w703 w789 w850 w1068 w1082 w1096 w1112]
      tunnel: [w53 w115 w181 w196 w294 w396 w559 w601 w703 w789 w846 w1068 w1082 w1096 w1112] -> w12
      tunnel: [_ _ _ _ _ w392 _ _ _ _ _ _ _ _ _] -> w11
      tunnel: w10 -> [_ _ _ _ _ _ _ _ _ _ _ _ _ _ _]
      tunnel: "Glue hehight" -> [_ _ _ _ _ _ _ _ w665 _ _ _ _ _ _]
      event "Inititalize": Value Change {
        (unwired) "INITIALIZING ....." ("String")
        (unwired) "ideal delta Y between \n2 fiducial marks"
        (unwired) "ideal delta X between 2 fiducial marks"
        # "center of lower module"
        # "center of upper module"
        n17 = event-data() -> ()  [unwired: 1 in, 6 out]
        n18 = Build Array(17.0 ("element"), 60.9 ("element"), 0.0 ("element"), 0.0 ("element")) -> (w77:dbl[])
        n19 = Build Array(17.0 ("element"), 411.0 ("element"), 0.0 ("element"), 0.0 ("element")) -> (w76:dbl[])
        n20 = case shown="True" w72 {
          tunnel: w77 -> [w97 w100]
          tunnel: w76 -> [w96 w99]
          tunnel: [w95 w98] -> w75
          frame False {
            n21 = Build Array(w96, w97) -> (w95:dbl[][])
          }
          frame True {
            n22 = Build Array(w100, w99) -> (w98:dbl[][])
          }
        }
        "default module position on stave" <- w75
        n23 = Build Array(24.3 ("y"), 231.4 ("y"), 0.0 ("element"), -0.05 ("element")) -> ()  [unwired: 1 out]
        n24 = Build Array(0.0 ("element"), 238.0 ("element"), 0.0 ("element"), 0.0 ("element")) -> (w59:dbl[])
        n25 = Add(x=w57, y=w59) -> (x+y=w58:dbl[])
        n26 = Build Array(w57, w58) -> (w56:dbl[][])
        n27 = for {
          N: 2 -> [_]
          tunnel: w69 -> [w94]
          tunnel: [w94] -> w67 mode=indexing
          tunnel: w68 -> [w93]
          tunnel: [w93] -> w66 mode=indexing
        }
        n28 = Index Array(array=w65, index=3) -> (element=w73:dbl)
        n29 = for {
          tunnel: w75 -> [w108] mode=indexing
          tunnel: w73 -> [w102]
          tunnel: w57 -> [w107]
          tunnel: [w105] -> _ mode=indexing
          (unwired) 0 ("index")
          n30 = Multiply(x=w102, y=-1.0) -> (x*y=w103:dbl)
          n31 = Index Array(array=w108) -> (element=w111:dbl)  [unwired: 1 in]
          n32 = Index Array(array=w108, index=1) -> (element=w110:dbl)
          n33 = call-poly <vilib>:"2D Cartesian Coordinate Rotation.vi"("theta"=w103, "y"=w110, "x"=w111) -> ("y out"=w113:dbl, "x out"=w112:dbl)  [unwired: 6 in, 1 out]
          n34 = Build Array(w112, w113, 0.0 ("element"), 0.0 ("element")) -> (w106:dbl[])
          n35 = Add(x=w106, y=w107) -> (x+y=w105:dbl[])
        }
      }
      event "Measure HDI": Value Change {
        (unwired) "HDI alignment in progress ..." ("String")
        n36 = event-data() -> ()  [unwired: 1 in, 6 out]
        n37 = for {
          N: w117 -> [_]
          tunnel: w126 -> [w143]
          shift-right: [w140] -> w128
          shift-left: w129 -> [w141]
          tunnel: w127 -> [w142]
          tunnel: [w177] -> w119 mode=indexing
          tunnel: [w176] -> w121 mode=indexing
          tunnel: [w130] -> w120 mode=indexing
          (unwired) "ideal delta Y between \n2 fiducial marks"
          (unwired) "ideal delta X between 2 fiducial marks"
          # "1"
          # "3"
          n38 = call "Joystick and Camera SHIH VPC- external Connection.vi"("Motion in"=w141, "XYZTheta"=w142, "Measurement Point"="Measure Top-Left of HDI") -> ("Motion out"=w156:refnum<class "Motion.lvclass">, "Sum"=w133:dbl[])  [unwired: 4 in, 2 out]
          n39 = Add(x=w143, y=w133) -> (x+y=w160:dbl[])
          n40 = Index Array(array=w133, index=0) -> (element=w147:dbl)
          n41 = Array Subset(array=w160, index=0, length=2) -> (w159:dbl[])
          n42 = Replace Array Subset(array=w159, new element=w147, index=0) -> (w157:dbl[])
          n43 = call-dynamic "XY Go.vi"("Speed"=100.0, "XY"=w157, "Motion in"=w156) -> ("Motion out"=w164:refnum<class "Motion.lvclass">)  [unwired: 7 in, 1 out]
          n44 = Build Array(24.3 ("y"), 231.4 ("y"), 0.0 ("element"), -0.05 ("element")) -> ()  [unwired: 1 out]
          n45 = call "Joystick and Camera SHIH VPC- external Connection.vi"("Motion in"=w164, "Measurement Point"="Measure Bottom-Left of HDI", "Inital GO"=FALSE) -> ("Motion out"=w155:refnum<class "Motion.lvclass">, "Sum"=w146:dbl[])  [unwired: 4 in, 2 out]
          n46 = Array Subset(array=w160, index=0, length=2) -> (w170:dbl[])
          n47 = Subtract(x=w146, y=w133) -> (x-y=w154:dbl[])
          n48 = call-dynamic "XY Go.vi"("Speed"=100.0, "XY"=w170, "Motion in"=w155) -> ("Motion out"=w174:refnum<class "Motion.lvclass">)  [unwired: 7 in, 1 out]
          n49 = call "XY_to_Rotation_RPHI.vi"("X-Y"=w154) -> ("r-phi"=w150:dbl[])
          n50 = call "Joystick and Camera SHIH VPC- external Connection.vi"("Motion in"=w174, "Measurement Point"="Measure Bottom-Righ of HDI", "Inital GO"=FALSE) -> ("Motion out"=w140:refnum<class "Motion.lvclass">, "Sum"=w137:dbl[])  [unwired: 4 in, 2 out]
          n51 = Subtract(x=w137, y=w133) -> (x-y=w138:dbl[])
          n52 = Index Array(array=w150, index=1) -> (element=w144:dbl)
          n53 = Multiply(x=w144, y=-1.0) -> (x*y=w135:dbl)
          n54 = Replace Array Subset(array=w138, new element=w135, index=3) -> (w176:dbl[])
          n55 = Replace Array Subset(array=w133, new element=w135, index=3) -> (w177:dbl[])
          n56 = Add(x=w137, y=w133) -> (x+y=w179:dbl[])
          n57 = Divide(x=w179, y=2.0) -> (x/y=w134:dbl[])
          n58 = Replace Array Subset(array=w134, new element=w135, index=3) -> (w131:dbl[])
          n59 = Subtract(x=w131, y=dbl[] [0.4, 0.4, 0.0, 0.0]) -> (x-y=w130:dbl[])
        }
      }
      event "Stop": Value Change {
        n60 = event-data() -> ()  [unwired: 1 in, 6 out]
        n61 = call "XYZTheta Go.vi"("XYZTheta In"=dbl[] [625.0, 625.0, 0.0, 0.01], "Motion in"=w195) -> ("Motion out"=w193:refnum<class "Motion.lvclass">)  [unwired: 7 in, 2 out]
      }
      event "Align Stave": Value Change {
        # "center of lower module"
        # "center of upper module"
        # "Default stave dimension\namong mounting holes"
        # "Measure 2 module positions on stave"
        n62 = event-data() -> ()  [unwired: 1 in, 6 out]
        n63 = Build Array(34.0 ("element"), 470.0 ("element"), 0.0 ("element"), 0.0 ("element")) -> ()  [unwired: 1 out]
        n64 = for {
          N: 1 -> [_]
          tunnel: w225 -> [w242]
          shift-right: [w252] -> w224
          shift-left: w227 -> [w253]
          tunnel: w226 -> [w254]
          tunnel: [w247] -> w200
          tunnel: [w245] -> w210
          (unwired) "ideal delta Y between \n2 fiducial marks"
          (unwired) "ideal delta X between 2 fiducial marks"
          n65 = call "Joystick and Camera SHIH VPC- external Connection.vi"("Motion in"=w253, "XYZTheta"=w254, "Measurement Point"="Measure Top-Left of stave") -> ("Motion out"=w236:refnum<class "Motion.lvclass">, "Sum"=w238:dbl[])  [unwired: 4 in, 2 out]
          n66 = Replace Array Subset(array=w242, new element=0.0 ("new element/subarray"), index=0) -> (w239:dbl[])
          n67 = Add(x=w238, y=w239) -> (x+y=w237:dbl[])
          n68 = call "Joystick and Camera SHIH VPC- external Connection.vi"("Motion in"=w236, "XYZTheta"=w237, "Measurement Point"="Measure Bottom-Left of stave", "Inital GO"=TRUE) -> ("Motion out"=w244:refnum<class "Motion.lvclass">, "Sum"=w257:dbl[])  [unwired: 3 in, 2 out]
          n69 = Build Array(24.3 ("y"), 231.4 ("y"), 0.0 ("element"), -0.05 ("element")) -> ()  [unwired: 1 out]
          n70 = Add(x=w242, y=w238) -> (x+y=w243:dbl[])
          n71 = Subtract(x=w257, y=w238) -> (x-y=w263:dbl[])
          n72 = call "XY_to_Rotation_RPHI.vi"("X-Y"=w263) -> ("r-phi"=w259:dbl[])
          n73 = Index Array(array=w259, index=1) -> (element=w255:dbl)
          n74 = call "Joystick and Camera SHIH VPC- external Connection.vi"("Motion in"=w244, "XYZTheta"=w243, "Measurement Point"="Measure Bottom-Righ of stave", "Inital GO"=TRUE) -> ("Motion out"=w252:refnum<class "Motion.lvclass">, "Sum"=w249:dbl[])  [unwired: 3 in, 2 out]
          n75 = Subtract(x=w249, y=w238) -> (x-y=w250:dbl[])
          n76 = Multiply(x=w255, y=-1.0) -> (x*y=w245:dbl)
          n77 = Replace Array Subset(array=w250, new element=w245, index=3) -> (→"measured stave size":dbl[])
          n78 = Replace Array Subset(array=w238, new element=w245, index=3) -> (w247:dbl[])
          n79 = Add(x=w249, y=w238) -> (x+y=w271:dbl[])
          n80 = Divide(x=w271, y=2.0) -> (x/y=→"Center of module on stave":dbl[])
        }
        n81 = Build Array(0.0 ("element"), 238.0 ("element"), 0.0 ("element"), 0.0 ("element")) -> (w201:dbl[])
        n82 = Add(x=w200, y=w201) -> (x+y=w199:dbl[])
        n83 = Build Array(w200, w199) -> (w198:dbl[][])
        n84 = Build Array(17.0 ("element"), 411.0 ("element"), 0.0 ("element"), 0.0 ("element")) -> (w212:dbl[])
        n85 = Build Array(17.0 ("element"), 60.9 ("element"), 0.0 ("element"), 0.0 ("element")) -> (w213:dbl[])
        n86 = case shown="True" w208 {
          tunnel: w213 -> [w290 w293]
          tunnel: w212 -> [w289 w292]
          tunnel: [w288 w291] -> w211
          frame False {
            n87 = Build Array(w289, w290) -> (w288:dbl[][])
          }
          frame True {
            n88 = Build Array(w293, w292) -> (w291:dbl[][])
          }
        }
        n89 = for {
          tunnel: w211 -> [w281] mode=indexing
          tunnel: w210 -> [w276]
          tunnel: w200 -> [w280]
          tunnel: [w278] -> w207 mode=indexing
          n90 = Multiply(x=w276, y=-1.0) -> (x*y=w275:dbl)
          n91 = Index Array(array=w281, index=0) -> (element=w284:dbl)
          n92 = Index Array(array=w281, index=1) -> (element=w283:dbl)
          n93 = call-poly <vilib>:"2D Cartesian Coordinate Rotation.vi"("theta"=w275, "y"=w283, "x"=w284) -> ("y out"=w286:dbl, "x out"=w285:dbl)  [unwired: 6 in, 1 out]
          n94 = Build Array(w285, w286, 0.0 ("element"), 0.0 ("element")) -> (w279:dbl[])
          n95 = Add(x=w279, y=w280) -> (x+y=w278:dbl[])
        }
      }
      event "Align Stave in detail": Value Change {
        # "center of lower module"
        # "center of upper module"
        # "Default stave dimension\namong mounting holes"
        # "Measure 2 module positions on stave"
        n96 = event-data() -> ()  [unwired: 1 in, 6 out]
        n97 = Build Array(34.0 ("element"), 470.0 ("element"), 0.0 ("element"), 0.0 ("element")) -> ()  [unwired: 1 out]
        n98 = for {
          N: 1 -> [_]
          tunnel: w323 -> [w340]
          shift-right: [w350] -> w322
          shift-left: w325 -> [w351]
          tunnel: w324 -> [w352]
          tunnel: [w345] -> w298
          tunnel: [w343] -> w308
          (unwired) "ideal delta Y between \n2 fiducial marks"
          (unwired) "ideal delta X between 2 fiducial marks"
          n99 = call "Joystick and Camera SHIH V5- external Connection.vi"("Motion in"=w351, "XYZTheta"=w352, "Measurement Point"="Measure Top-Left of stave") -> ("final out"=w336:dbl[], "Motion out"=w334:refnum<class "Motion.lvclass">)  [unwired: 5 in, 1 out]
          n100 = Replace Array Subset(array=w340, new element=0.0 ("new element/subarray"), index=0) -> (w337:dbl[])
          n101 = Add(x=w336, y=w337) -> (x+y=w335:dbl[])
          n102 = call "Joystick and Camera SHIH V5- external Connection.vi"("Motion in"=w334, "XYZTheta"=w335, "Measurement Point"="Measure Bottom-Left of stave", "Inital GO"=TRUE) -> ("final out"=w355:dbl[], "Motion out"=w342:refnum<class "Motion.lvclass">)  [unwired: 4 in, 1 out]
          n103 = Build Array(24.3 ("y"), 231.4 ("y"), 0.0 ("element"), -0.05 ("element")) -> ()  [unwired: 1 out]
          n104 = Add(x=w340, y=w336) -> (x+y=w341:dbl[])
          n105 = Subtract(x=w355, y=w336) -> (x-y=w361:dbl[])
          n106 = call "XY_to_Rotation_RPHI.vi"("X-Y"=w361) -> ("r-phi"=w357:dbl[])
          n107 = Index Array(array=w357, index=1) -> (element=w353:dbl)
          n108 = call "Joystick and Camera SHIH V5- external Connection.vi"("Motion in"=w342, "XYZTheta"=w341, "Measurement Point"="Measure Bottom-Righ of stave", "Inital GO"=TRUE) -> ("final out"=w347:dbl[], "Motion out"=w350:refnum<class "Motion.lvclass">)  [unwired: 4 in, 1 out]
          n109 = Subtract(x=w347, y=w336) -> (x-y=w348:dbl[])
          n110 = Multiply(x=w353, y=-1.0) -> (x*y=w343:dbl)
          n111 = Replace Array Subset(array=w348, new element=w343, index=3) -> (→"FROM Detail !! measured stave size":dbl[])
          n112 = Replace Array Subset(array=w336, new element=w343, index=3) -> (w345:dbl[])
          n113 = Add(x=w347, y=w336) -> (x+y=w369:dbl[])
          n114 = Divide(x=w369, y=2.0) -> (x/y=→"FROM Detail !!! Center of module on stave":dbl[])
        }
        n115 = Build Array(0.0 ("element"), 238.0 ("element"), 0.0 ("element"), 0.0 ("element")) -> (w299:dbl[])
        n116 = Add(x=w298, y=w299) -> (x+y=w297:dbl[])
        n117 = Build Array(w298, w297) -> (w296:dbl[][])
        n118 = Build Array(17.0 ("element"), 411.0 ("element"), 0.0 ("element"), 0.0 ("element")) -> (w310:dbl[])
        n119 = Build Array(17.0 ("element"), 60.9 ("element"), 0.0 ("element"), 0.0 ("element")) -> (w311:dbl[])
        n120 = case shown="True" w306 {
          tunnel: w311 -> [w388 w391]
          tunnel: w310 -> [w387 w390]
          tunnel: [w386 w389] -> w309
          frame False {
            n121 = Build Array(w387, w388) -> (w386:dbl[][])
          }
          frame True {
            n122 = Build Array(w391, w390) -> (w389:dbl[][])
          }
        }
        n123 = for {
          tunnel: w309 -> [w379] mode=indexing
          tunnel: w308 -> [w374]
          tunnel: w298 -> [w378]
          tunnel: [w376] -> w305 mode=indexing
          n124 = Multiply(x=w374, y=-1.0) -> (x*y=w373:dbl)
          n125 = Index Array(array=w379, index=0) -> (element=w382:dbl)
          n126 = Index Array(array=w379, index=1) -> (element=w381:dbl)
          n127 = call-poly <vilib>:"2D Cartesian Coordinate Rotation.vi"("theta"=w373, "y"=w381, "x"=w382) -> ("y out"=w384:dbl, "x out"=w383:dbl)  [unwired: 6 in, 1 out]
          n128 = Build Array(w383, w384, 0.0 ("element"), 0.0 ("element")) -> (w377:dbl[])
          n129 = Add(x=w377, y=w378) -> (x+y=w376:dbl[])
        }
      }
      event "Bless from OGP": Value Change {
        # "center of upper module"
        # "center of lower module"
        # "center of upper module"
        # "NL line with correct rotation"
        # "Default stave dimension\namong mounting holes"
        # "Measure 2 module positions on stave"
        n130 = event-data() -> ()  [unwired: 1 in, 6 out]
        n131 = Build Array(34.0 ("element"), 470.0 ("element"), 0.0 ("element"), 0.0 ("element")) -> ()  [unwired: 1 out]
        n132 = for {
          N: 1 -> [_]
          tunnel: w444 -> [_]
          shift-right: [w504] -> w443
          shift-left: w427 -> [w517]
          tunnel: w429 -> [_]
          tunnel: [w496] -> w432
          tunnel: [w499] -> w440
          tunnel: w428 -> [w506]
          tunnel: [w482] -> w392
          (unwired) FALSE ("Inital GO")
          (unwired) "ideal delta Y between \n2 fiducial marks"
          (unwired) "ideal delta X between 2 fiducial marks"
          # "after NL"
          # "after SL"
          # "NL line"
          # "rotation"
          n133 = call "Joystick and Camera SHIH VPC- external Connection.vi"("Motion in"=w517, "XYZTheta"=dbl[] [576.333, 663.131, 70.7812, 0.010000094994154989] ("N chip"), "Measurement Point"="north chip", "Inital GO"=TRUE) -> ("Motion out"=w514:refnum<class "Motion.lvclass">, "Sum"=w494:dbl[])  [unwired: 3 in, 2 out]
          "N chip" <- w494
          n134 = call "Joystick and Camera SHIH VPC- external Connection.vi"("Motion in"=w514, "XYZTheta"=dbl[] [578.791, 1154.64, 70.5935, 0.010000670236950445] ("S chip"), "Measurement Point"="south chip", "Inital GO"=TRUE) -> ("Motion out"=w513:refnum<class "Motion.lvclass">, "Sum"=w495:dbl[])  [unwired: 3 in, 2 out]
          "S chip" <- w495
          n135 = Subtract(x=w495, y=w494) -> (x-y=w493:dbl[])
          n136 = Index Array(array=w493, index #1=0 ("index"), index #2=1 ("index")) -> (element #1=w490:dbl, element #2=w489:dbl)
          n137 = Square(x=w490) -> (x^2=w487:dbl)
          n138 = Square(x=w489) -> (x^2=w488:dbl)
          n139 = Add(x=w487, y=w488) -> (x+y=w486:dbl)
          n140 = call "Joystick and Camera SHIH VPC- external Connection.vi"("Motion in"=w513, "Measurement Point"="height of stave", "Inital GO"=FALSE) -> ("Motion out"=w504:refnum<class "Motion.lvclass">, "Sum"=w505:dbl[])  [unwired: 4 in, 2 out]
          n141 = call "O to G peek.vi"("height"=w505, "south chip"=w495, "north chip"=w494, "Input file"=w506) -> ("OGP length"=→"chip distance by OGP":dbl, "output BR"=w508:dbl[], "output BL"=w507:dbl[], "output TL"=w501:dbl[])  [unwired: 4 in]
          "after NL" <- w501
          "after SR" <- w508
          "after SL" <- w507
          n142 = Square Root(x=w486) -> (sqrt(x)=→"chip distance by gantry":dbl)
          n143 = Subtract(x=w508, y=w501) -> (x-y=w519:dbl[])
          n144 = Build Array(24.3 ("y"), 231.4 ("y"), 0.0 ("element"), -0.05 ("element")) -> ()  [unwired: 1 out]
          n145 = Subtract(x=w507, y=w501) -> (x-y=w525:dbl[])
          n146 = call "XY_to_Rotation_RPHI.vi"("X-Y"=w525) -> ("r-phi"=w524:dbl[])
          n147 = Index Array(array=w524, index=1) -> (element=w521:dbl)
          n148 = Multiply(x=w521, y=-1.0) -> (x*y=w499:dbl)
          n149 = Replace Array Subset(array=w519, new element=w499, index=3) -> (→"bless from OGP !! measured stave size":dbl[])
          n150 = Replace Array Subset(array=w501, new element=w499, index=3) -> (w497:dbl[])
          n151 = Add(x=w508, y=w501) -> (x+y=w531:dbl[])
          n152 = Divide(x=w531, y=2.0) -> (x/y=w483:dbl[])
          n153 = Add(x=w497, y=dbl[] [0.0, 10.0, 0.0, 0.0]) -> (x+y=w496:dbl[])
          n154 = Replace Array Subset(array=w483, new element=w499, index=3) -> (w482:dbl[])
          "bless from OGP !!! Center of  stave" <- w482
        }
        n155 = Build Array(0.0 ("element"), 238.0 ("element"), 0.0 ("element"), 0.0 ("element")) -> (w433:dbl[])
        n156 = Add(x=w432, y=w433) -> (x+y=w431:dbl[])
        n157 = Build Array(w432, w431) -> (w430:dbl[][])
        n158 = Build Array(0.0 ("element"), 116.65 ("element"), 0.0 ("element"), 0.0 ("element")) -> (w416:dbl[])
        n159 = Build Array(0.0 ("element"), -116.65 ("element"), 0.0 ("element"), 0.0 ("element")) -> (w417:dbl[])
        n160 = Build Array(0.0 ("element"), 116.65 ("element"), 0.0 ("element"), 0.0 ("element")) -> (w399:dbl[])
        n161 = Build Array(0.0 ("element"), -116.65 ("element"), 0.0 ("element"), 0.0 ("element")) -> (w400:dbl[])
        n162 = case shown="True" w398 {
          tunnel: w417 -> [w478 w481]
          tunnel: w416 -> [w477 w480]
          tunnel: [w476 w479] -> w415
          frame False {
            n163 = Build Array(w477, w478) -> (w476:dbl[][])
          }
          frame True {
            n164 = Build Array(w481, w480) -> (w479:dbl[][])
          }
        }
        n165 = case shown="True" w398 {
          tunnel: w400 -> [w455 w458]
          tunnel: w399 -> [w454 w457]
          tunnel: [w453 w456] -> w397
          frame False {
            n166 = Build Array(w454, w455) -> (w453:dbl[][])
          }
          frame True {
            n167 = Build Array(w458, w457) -> (w456:dbl[][])
          }
        }
        n168 = for {
          tunnel: w415 -> [w552] mode=indexing
          tunnel: w440 -> [w549]
          tunnel: [w551] -> w426 mode=indexing
          tunnel: w392 -> [w534]
          tunnel: [w546] -> w414 mode=indexing
          tunnel: w397 -> [w537] mode=indexing
          tunnel: [w533] -> w395 mode=indexing
          n169 = Multiply(x=w549, y=-1.0) -> (x*y=w536:dbl)
          n170 = Index Array(array=w552, index=0) -> (element=w555:dbl)
          n171 = Index Array(array=w552, index=1) -> (element=w554:dbl)
          n172 = Index Array(array=w537, index=0) -> (element=w542:dbl)
          n173 = Index Array(array=w537, index=1) -> (element=w541:dbl)
          n174 = call-poly <vilib>:"2D Cartesian Coordinate Rotation.vi"("theta"=w536, "y"=w554, "x"=w555) -> ("y out"=w557:dbl, "x out"=w556:dbl)  [unwired: 6 in, 1 out]
          n175 = call-poly <vilib>:"2D Cartesian Coordinate Rotation.vi"("theta"=w536, "y"=w541, "x"=w542) -> ("y out"=w544:dbl, "x out"=w543:dbl)  [unwired: 6 in, 1 out]
          n176 = Build Array(w556, w557, 0.0 ("element"), 0.0 ("element")) -> (w546:dbl[])
          n177 = Build Array(w543, w544, 0.0 ("element"), 0.0 ("element")) -> (w535:dbl[])
          n178 = Add(x=w535, y=w534) -> (x+y=w533:dbl[])
          n179 = Add(x=w546, y=w534) -> (x+y=w551:dbl[])
        }
        "CT HPoS" <- w414
        "HDI center positions" <- w395
        n180 = Add(x=w426, y=w413) -> (x+y=w412:dbl[][])
        n181 = call-poly <vilib>:"Write Delimited Spreadsheet.vi"("file path (dialog if empty)"=path "D:/INTT/V1/Assembly Data/ladder assembly/2line_switch.txt", "format (%.3f)"="%.10f", "2D data"=w412) -> ()  [unwired: 11 in, 2 out]
        n182 = disable-structure shown="Disabled" {
          disable-tunnel: w398 -> [w459 _]
          frame Disabled {
            # "center of lower module"
            # "center of upper module"
            n183 = Build Array(17.0 ("element"), 60.9 ("element"), 0.0 ("element"), 0.0 ("element")) -> (w461:dbl[])
            n184 = Build Array(17.0 ("element"), 411.0 ("element"), 0.0 ("element"), 0.0 ("element")) -> (w460:dbl[])
            n185 = case shown="True" w459 {
              tunnel: w461 -> [w472 w475]
              tunnel: w460 -> [w471 w474]
              tunnel: [w470 w473] -> _
              frame False {
                n186 = Build Array(w471, w472) -> (w470:dbl[][])
              }
              frame True {
                n187 = Build Array(w475, w474) -> (w473:dbl[][])
              }
            }
          }
          frame Enabled {
          }
        }
        n188 = call-poly <vilib>:"Write Delimited Spreadsheet.vi"("file path (dialog if empty)"=path "D:/INTT/V1/Assembly Data/ladder assembly/stave_HDI_center.txt", "format (%.3f)"="%.8f", "2D data"=w395) -> ()  [unwired: 11 in, 2 out]
      }
      event "txt switch": Value Change {
        n189 = event-data() -> ()  [unwired: 1 in, 6 out]
        n190 = flat-sequence {
          tunnel: [w581] -> w575
          tunnel: w565 -> [w577]
          tunnel: [w577] -> w564
          tunnel: w562 -> [w576]
          tunnel: [w576] -> w561
          tunnel: w575 -> [w599]
          tunnel: [w597] -> w563
          tunnel: w564 -> [w597]
          tunnel: [w596] -> w560
          tunnel: w561 -> [w596]
          frame #0 {
            n191 = call-poly <vilib>:"Read Delimited Spreadsheet.vi"("file path (dialog if empty)"=path "D:/INTT/V1/Assembly Data/ladder assembly/2line_switch.txt" ("file path (dialog if empty) 3"), "format (%.3f)"="%.10f") -> ("all rows"=w582:dbl[][])  [unwired: 8 in, 5 out]
            n192 = Array Subset(array=w582, index (row)=0 ("index"), length (row)=1 ("length"), index (col)=0 ("index"), length (col)=4 ("length")) -> (w592:dbl[][])
            n193 = Reshape Array(w592, 4 ("dimension size")) -> (w579:dbl[])
            n194 = Array Subset(array=w582, index (row)=1 ("index"), length (row)=1 ("length"), index (col)=0 ("index"), length (col)=4 ("length")) -> (w586:dbl[][])
            n195 = Reshape Array(w586, 4 ("dimension size")) -> (w580:dbl[])
            n196 = Build Array(w580, w579) -> (w581:dbl[][])
          }
          frame #1 {
            n197 = call-poly <vilib>:"Write Delimited Spreadsheet.vi"("file path (dialog if empty)"=path "D:/INTT/V1/Assembly Data/ladder assembly/2line_switch.txt" ("file path (dialog if empty) 4"), "format (%.3f)"="%.10f", "2D data"=w599) -> ()  [unwired: 11 in, 2 out]
          }
        }
      }
      event "Measure Pickup Tools": Value Change {
        (unwired) "Measuring Pickup Tools" ("String")
        n198 = event-data() -> ()  [unwired: 1 in, 6 out]
        n199 = for {
          N: w602 -> [_]
          tunnel: [w638] -> w613 mode=indexing
          tunnel: w614 -> [w642]
          tunnel: [w624] -> w612
          tunnel: w611 -> [w623] mode=indexing
          # "Default size and\norientation"
          n200 = call "Joystick and Camera SHIH VPC- external Connection.vi"("Motion in"=w642, "XYZTheta"=w623, "Measurement Point"="PickUp tool Top") -> ("Motion out"=w618:refnum<class "Motion.lvclass">, "Sum"=w641:dbl[])  [unwired: 4 in, 2 out]
          n201 = Build Array(0.0 ("element"), 29.94 ("element"), 0.0 ("element"), 0.0 ("element")) -> (w629:dbl[])
          n202 = Add(x=w641, y=w629) -> (x+y=w615:dbl[])
          n203 = Array Subset(array=w615, index=0, length=2) -> (w616:dbl[])
          n204 = call-dynamic "XY Go.vi"("Speed"=20.0, "XY"=w616, "Motion in"=w618) -> ("Motion out"=w617:refnum<class "Motion.lvclass">)  [unwired: 7 in, 1 out]
          n205 = call "Joystick and Camera SHIH VPC- external Connection.vi"("Motion in"=w617, "Measurement Point"="PickUp tool Bottom", "Inital GO"=FALSE) -> ("Motion out"=w624:refnum<class "Motion.lvclass">, "Sum"=w640:dbl[])  [unwired: 4 in, 2 out]
          n206 = Add(x=w641, y=w640) -> (x+y=w647:dbl[])
          n207 = Subtract(x=w640, y=w641) -> (x-y=w639:dbl[])
          n208 = Divide(x=w647, y=2.0) -> (x/y=w644:dbl[])
          n209 = call "XYtoRPHI.vi"("X-Y"=w639) -> ("r-phi"=w645:dbl[])
          n210 = Index Array(array=w645, index=1) -> (element=w633:dbl)
          n211 = Absolute Value(x=w633) -> (abs(x)=w636:dbl)
          n212 = Sign(1:w633) -> (0:w634:dbl)
          n213 = Subtract(x=w636, y=1.5707963267948966) -> (x-y=w635:dbl)
          n214 = Multiply(x=w634, y=w635) -> (x*y=w632:dbl)
          n215 = Replace Array Subset(array=w644, new element=w632, index=3) -> (w638:dbl[])
          "PickupTool \nCenterPosition" <- w638
        }
      }
      event "Deposit Glue": Value Change {
        w653 = 20.0 ("Speed")
        # "CF height"
        # "surface z offset"
        # "two sensor, Sensor B then A"
        # "Unmount syringe"
        # "first needle park position\nneedle gap on Z value : 0.5 mm"
        # "Syringe-camera offset"
        n216 = event-data() -> ()  [unwired: 1 in, 6 out]
        n217 = call-poly <vilib>:"Read Delimited Spreadsheet.vi"("file path (dialog if empty)"=path "D:/INTT/V1/Assembly Data/Tool Offsets/Dispense Tip Offset.txt", "number of rows (all:-1)"=-1) -> ("first row"=w747:dbl[])  [unwired: 8 in, 5 out]
        n218 = Add(x=14.2 ("element"), y=w713) -> (x+y=w709:dbl)
        n219 = Add(x=70.9882 ("y"), y=w709) -> (x+y=w708:dbl)
        n220 = Build Array(427.051, 722.276, w708, 0.0 ("element")) -> (w707:dbl[])
        "Needle parking position" <- w707
        n221 = Index Array(array=w747, index #1=0 ("index"), index #2=1 ("index")) -> (element #1=w704:dbl, element #2=w741:dbl)
        n222 = Build Array(w704, w741, 0.0 ("element"), 0.0 ("element")) -> (w699:dbl[])
        n223 = call "XYZTheta Go.vi"("XYZTheta In"=w707, "Motion in"=w736) -> ("error out"=w740:errorcluster, "Motion out"=w735:refnum<class "Motion.lvclass">)  [unwired: 7 in, 1 out]
        n224 = call "Display Message to User"("error in (no error)"=w740) -> ("error out"=w737:errorcluster)  [unwired: 9 in, 1 out]
        n225 = Array Subset(array=w706, index (row)=0, length (row)=1 ("length")) -> (w714:dbl[][])  [unwired: 2 in]
        n226 = Reshape Array(w714, 4 ("dimension size")) -> (w711:dbl[])
        n227 = Index Array(array=w711, index=2) -> ()  [unwired: 1 out]
        n228 = case shown="False" w712 {
          tunnel: w706 -> [w779 w788]
          tunnel: [w776 w788] -> w660
          frame False {
            n229 = Array Subset(array=w779, index (row)=1 ("index"), length (row)=1 ("length")) -> (w780:dbl[][])  [unwired: 2 in]
            n230 = Array Subset(array=w779, index (row)=0 ("index"), length (row)=1 ("length")) -> (w783:dbl[][])  [unwired: 2 in]
            n231 = Reshape Array(w783, 4 ("dimension size")) -> (w778:dbl[])
            n232 = Reshape Array(w780, 4 ("dimension size")) -> (w777:dbl[])
            n233 = Build Array(w777, w778) -> (w776:dbl[][])
          }
          frame True {
          }
        }
        n234 = call-dynamic "Z Go.vi"("error in (no error)"=w737, "Speed"=20.0, "Position"=0.0, "Motion in"=w735) -> ("error out"=w734:errorcluster, "Motion out"=w702:refnum<class "Motion.lvclass">)  [unwired: 6 in]
        n235 = call "Display Message to User2"("error in (no error)"=w734) -> ("error out"=w701:errorcluster)  [unwired: 9 in, 1 out]
        n236 = Add(x=dbl[] [3.3, 5.0, 0.0, 0.0] ("y"), y=dbl[] [13.7, 15.0, 0.0, 0.0]) -> (x+y=w675:dbl[])
        n237 = Array Subset(array=w660, index (row)=0 ("index"), length (row)=1 ("length")) -> (w696:dbl[][])  [unwired: 2 in]
        n238 = Reshape Array(w696, 4 ("dimension size")) -> (w694:dbl[])
        "output array" <- w694
        n239 = Add(x=w694, y=w699) -> (x+y=w678:dbl[])
        n240 = Add(x=w678, y=w675) -> (x+y=w679:dbl[])
        n241 = Array Subset(array=w679, index=0, length=2) -> (w674:dbl[])
        n242 = call-dynamic "Connect.vi"("Ultimus V in"=refnum<class "Ultimus V2.lvclass"> refnum ("Ultimus V2.lvclass")) -> ("Ultimus V out"=w733:refnum<class "Ultimus V2.lvclass">)  [unwired: 9 in, 1 out]
        n243 = Index Array(array=w694, index=2) -> (element=w667:dbl)
        n244 = Array Subset(array=w660, index (row)=1 ("index"), length (row)=1 ("length")) -> (w662:dbl[][])  [unwired: 2 in]
        n245 = Reshape Array(w662, 4 ("dimension size")) -> (w658:dbl[])
        n246 = call-dynamic "XY Go.vi"("error in (no error)"=w701, "Speed"=100.0, "XY"=w674, "Motion in"=w702) -> ("error out"=w684:errorcluster, "Motion out"=w685:refnum<class "Motion.lvclass">)  [unwired: 6 in]
        n247 = Subtract(x=5.5818 ("y"), y=w665) -> (x-y=w669:dbl)
        n248 = Add(x=w667, y=w669) -> (x+y=w666:dbl)
        n249 = Add(x=w666, y=-2.0) -> (x+y=w686:dbl)
        n250 = call-dynamic "Z Go.vi"("error in (no error)"=w684, "Speed"=5.0, "Position"=w686, "Motion in"=w685) -> ("error out"=w650:errorcluster, "Motion out"=w683:refnum<class "Motion.lvclass">)  [unwired: 6 in]
        n251 = flat-sequence {
          tunnel: w733 -> [w767]
          tunnel: [w767] -> w693
          tunnel: [w766] -> w692
          tunnel: [w765] -> w691
          tunnel: w693 -> [w775]
          tunnel: [w774] -> w700
          tunnel: [w769] -> _
          tunnel: w692 -> [w770]
          tunnel: w691 -> [w769]
          tunnel: w683 -> [w773]
          tunnel: [w772] -> w652
          tunnel: dbl[][] [[0.0, 194.0]] ("distances") -> [w771]
          frame #0 {
            n252 = call "air pressure setting.vi"() -> ("air pressure indecator"=w765:i32, "deposit speed 2"=w766:dbl)
          }
          frame #1 {
            n253 = call "Muliti_XY_dispense.vi"("Pressure"=w769, "Path count"=1, "Speed"=w770, "distances"=w771, "Ultimus V in"=w775, "Motion in"=w773) -> ("Ultimus V out"=w774:refnum<class "Ultimus V2.lvclass">, "Motion out"=w772:refnum<class "Motion.lvclass">)  [unwired: 4 in]
          }
        }
        n254 = Add(x=w658, y=dbl[] [17.0, 20.0, 0.0, 0.0]) -> (x+y=w657:dbl[])
        n255 = disable-structure shown="Disabled" {
          disable-tunnel: w657 -> [w753 _]
          disable-tunnel: w653 -> [w752 _]
          frame Disabled {
            n256 = call-dynamic "XY Go.vi"("Speed"=w752, "XY"=w753) -> ()  [unwired: 8 in, 2 out]
          }
          frame Enabled {
          }
        }
        n257 = call-dynamic "wrtCurrent Go.vi"("axis names"=string[] ["X", "Y"], "error in (no error)"=w650, "Speed"=w653, "distances"=dbl[] [0.0, 44.0], "Motion in"=w652) -> ("error out"=w649:errorcluster, "Motion out"=w651:refnum<class "Motion.lvclass">)  [unwired: 5 in]
        n258 = flat-sequence {
          tunnel: w700 -> [w756]
          tunnel: [w756] -> w673
          tunnel: [w755] -> w672
          tunnel: [w754] -> w671
          tunnel: w673 -> [w764]
          tunnel: [w763] -> w720
          tunnel: w672 -> [w762]
          tunnel: w671 -> [w757]
          tunnel: w651 -> [w761]
          tunnel: [w760] -> w721
          tunnel: dbl[][] [[0.0, 194.0]] ("distances") -> [w758]
          frame #0 {
            n259 = call "air pressure setting.vi"() -> ("air pressure indecator"=w754:i32, "deposit speed 2"=w755:dbl)
          }
          frame #1 {
            n260 = call "Muliti_XY_dispense.vi"("Pressure"=w757, "Path count"=1, "Speed"=w762, "distances"=w758, "Ultimus V in"=w764, "Motion in"=w761) -> ("Ultimus V out"=w763:refnum<class "Ultimus V2.lvclass">, "Motion out"=w760:refnum<class "Motion.lvclass">)  [unwired: 4 in]
          }
        }
        n261 = call "XYZTheta Go.vi"("error in (no error)"=w649, "XYZTheta In"=dbl[] [500.0, 1000.0, 0.0, 0.1], "Motion in"=w721) -> ("error out"=w731:errorcluster, "Motion out"=w729:refnum<class "Motion.lvclass">)  [unwired: 6 in, 1 out]
        n262 = call-dynamic "Disconnect.vi"("Ultimus V in"=w720) -> ()  [unwired: 9 in, 1 out]
        n263 = call "Display Message to User3"("error in (no error)"=w731) -> ()  [unwired: 9 in, 2 out]
      }
      event "Needle Alignment": Value Change {
        (unwired) "Needle Alignment in progress ...." ("String")
        # "CF height"
        # "surface z offset"
        # "first needle park position\nneedle gap on Z value : 0.5 mm"
        # "Syringe-camera offset"
        n264 = event-data() -> ()  [unwired: 1 in, 6 out]
        n265 = Array Subset(array=w792, index (row)=0, length (row)=1 ("length")) -> (w795:dbl[][])  [unwired: 2 in]
        n266 = Reshape Array(w795, 4 ("dimension size")) -> (w794:dbl[])
        n267 = Index Array(array=w794, index=2) -> (element=w791:dbl)
        n268 = call-poly <vilib>:"Read Delimited Spreadsheet.vi"("file path (dialog if empty)"=path "D:/INTT/V1/Assembly Data/Tool Offsets/Dispense Tip Offset.txt", "number of rows (all:-1)"=-1) -> ("first row"=w842:dbl[])  [unwired: 8 in, 5 out]
        n269 = Index Array(array=w842, index #1=0 ("index"), index #2=1 ("index")) -> (element #1=w837:dbl, element #2=w836:dbl)
        n270 = Add(x=14.2 ("element"), y=w800) -> (x+y=w802:dbl)
        n271 = Add(x=w791, y=w802) -> (x+y=w801:dbl)
        n272 = Build Array(424.448, 1040.76, w801, 0.0 ("element")) -> (w799:dbl[])
        n273 = Build Array(w837, w836, 0.0 ("element"), 0.0 ("element")) -> (w811:dbl[])
        n274 = call "XYZTheta Go.vi"("XYZTheta In"=w799, "Motion in"=w826) -> ("error out"=w835:errorcluster, "XYZTheta Out"=w816:dbl[], "Motion out"=w825:refnum<class "Motion.lvclass">)  [unwired: 7 in]
        n275 = call "Display Message to User10"("error in (no error)"=w835) -> ("error out"=w832:errorcluster)  [unwired: 9 in, 1 out]
        n276 = call-dynamic "Z Go.vi"("error in (no error)"=w832, "Speed"=20.0, "Position"=0.0, "Motion in"=w825) -> ("Motion out"=w824:refnum<class "Motion.lvclass">)  [unwired: 6 in, 1 out]
        n277 = Replace Array Subset(array=w816, new element=0.0 ("new element/subarray"), index=2) -> (w813:dbl[])
        n278 = call "Joystick and Camera SHIH VPC- external Connection.vi"("Motion in"=w824, "XYZTheta"=w813, "Measurement Point"="Touch Needle on a surface") -> ("Motion out"=w822:refnum<class "Motion.lvclass">, "Gantry"=w812:dbl[])  [unwired: 4 in, 2 out]
        n279 = Subtract(x=w812, y=w811) -> (x-y=w810:dbl[])
        n280 = call "Joystick and Camera SHIH VPC- external Connection.vi"("Motion in"=w822, "XYZTheta"=w810, "Measurement Point"="Measure the touch spot with camera") -> ("Motion out"=w818:refnum<class "Motion.lvclass">, "Gantry"=w821:dbl[])  [unwired: 4 in, 2 out]
        n281 = Subtract(x=w812, y=w821) -> (x-y=w820:dbl[])
        n282 = call-poly <vilib>:"Write Delimited Spreadsheet.vi"("file path (dialog if empty)"=path "D:/INTT/V1/Assembly Data/Tool Offsets/Dispense Tip Offset.txt", "1D data"=w820, "append to file? (new file:F)"=FALSE) -> ()  [unwired: 11 in, 2 out]
      }
      event "Pick and place": Value Change {
        (unwired) "PICK and PLACE samples ..." ("String")
        n283 = event-data() -> ()  [unwired: 1 in, 6 out]
        n284 = Build Array(0.0 ("element"), 0.0 ("element"), 0.0 ("element"), 0.0 ("element")) -> (w860:dbl[])
        n285 = Build Array(0.0 ("element"), 0.0 ("element"), 0.0 ("element"), 0.0 ("element")) -> (w859:dbl[])
        n286 = case shown="False" w854 {
          tunnel: w879 -> [w1045 w1067]
          tunnel: [w1044 w1066] -> _
          frame False {
            n287 = Array Subset(array=w1045, index (row)=0 ("index"), length (row)=1 ("length")) -> (w1047:dbl[][])  [unwired: 2 in]
            n288 = Build Array(11.75 ("element"), 173.55 ("element"), 0.0 ("element"), 0.0 ("element")) -> (w1051:dbl[])
            n289 = Reshape Array(w1047, 4 ("dimension size")) -> (w1046:dbl[])
            n290 = Add(x=w1051, y=w1046) -> (x+y=w1044:dbl[])
          }
          frame True {
            n291 = Array Subset(array=w1067, index (row)=0 ("index"), length (row)=1 ("length")) -> (w1057:dbl[][])  [unwired: 2 in]
            n292 = Build Array(11.75 ("element"), 56.85 ("element"), 0.0 ("element"), 0.0 ("element")) -> (w1061:dbl[])
            n293 = Reshape Array(w1057, 4 ("dimension size")) -> (w1056:dbl[])
            n294 = Add(x=w1061, y=w1056) -> (x+y=w1066:dbl[])
          }
        }
        n295 = Not(x=w854) -> (.not. x?=w853:bool)
        n296 = case shown="True" w853 {
          tunnel: w860 -> [w1038 w1041]
          tunnel: w859 -> [w1039 w1042]
          tunnel: [w1040 w1043] -> w858
          frame False {
            n297 = Build Array(w1039, w1038) -> (w1040:dbl[][])
          }
          frame True {
            n298 = Build Array(w1041, w1042) -> (w1043:dbl[][])
          }
        }
        n299 = Add(x=1.0, y=w850) -> (x+y=w846:dbl)
        n300 = Quotient & Remainder(x=w846, y=2.0) -> (x-y*floor(x/y)=w848:dbl)  [unwired: 1 out]
        n301 = Equal To 0?(x=w848) -> (x = 0?=w847:bool)
        n302 = for {
          tunnel: [w903] -> w852
          tunnel: w858 -> [w902] mode=indexing
          tunnel: w855 -> [w899] mode=indexing
          n303 = Index Array(array=w899, index=3) -> (element=w900:dbl)
          n304 = Multiply(x=w900, y=-1.0) -> (x*y=w898:dbl)
          n305 = Index Array(array=w902, index=0) -> (element=w909:dbl)
          n306 = Index Array(array=w902, index=1) -> (element=w908:dbl)
          n307 = call-poly <vilib>:"2D Cartesian Coordinate Rotation.vi"("theta"=w898, "y"=w908, "x"=w909) -> ("y out"=w911:dbl, "x out"=w910:dbl)  [unwired: 6 in, 1 out]
          n308 = Build Array(w910, w911, 0.0 ("element"), 0.0 ("element")) -> (w903:dbl[])
        }
        "?" <- w852
        n309 = Array Subset(array=w855, index (row)=0 ("index"), length (row)=1 ("length")) -> (w866:dbl[][])  [unwired: 2 in]
        n310 = Reshape Array(w866, 4 ("dimension size")) -> (w857:dbl[])
        n311 = Add(x=w852, y=w857) -> (x+y=w856:dbl[])
        "CT sum up" <- w856
        n312 = call-poly <vilib>:"Read Delimited Spreadsheet.vi"("file path (dialog if empty)"=path "D:/INTT/V1/Assembly Data/Tool Offsets/Bellows Tool Offset.txt", "number of rows (all:-1)"=-1) -> ("first row"=w894:dbl[])  [unwired: 8 in, 5 out]
        n313 = Index Array(array=w894, index #1=0 ("index"), index #2=1 ("index"), index #3=2 ("index")) -> (element #1=w890:dbl, element #2=w889:dbl, element #3=w888:dbl)
        n314 = for {
          N: 1 -> [_]
          tunnel: w897 -> [w927]
          tunnel: [w947] -> w887
          tunnel: w886 -> [w921] mode=indexing
          tunnel: [w935] -> w882
          tunnel: w883 -> [w926]
          tunnel: w890 -> [w949]
          tunnel: w889 -> [w948]
          tunnel: w888 -> [w946]
          tunnel: w875 -> [w941]
          tunnel: w881 -> [w929]
          tunnel: w856 -> [w928]
          tunnel: w877 -> [w924]
          tunnel: w855 -> [w920]
          tunnel: w852 -> [w919]
          tunnel: w847 -> [w918]
          w937 = 0 ("Write")
          w940 = TRUE ("Write Value")
          # "putback pickup tool"
          # "pickup tool"
          # "pickup tool height offset"
          # "Pick up PICKUP TOOL"
          # "Pick up CHIPs/Sensor and place on HDI"
          n315 = Build Array(w949, w948, w946, 0.0 ("element")) -> (w922:dbl[])
          n316 = Add(x=w921, y=w922) -> (x+y=w916:dbl[])
          n317 = call "XYZTheta-2Zspeed Go.vi"("XYZTheta In"=w916, "Motion in"=w927) -> ("error out"=w925:errorcluster, "Motion out"=w923:refnum<class "Motion.lvclass">)  [unwired: 7 in, 1 out]
          n318 = call "WriteReadWait.vi"("Read Value"=w940, "Write Value"=w940, "error in (no error)"=w925, "Read"=w937, "Write"=w937, "I-O in"=w926) -> ("error out"=w939:errorcluster, "I-O out"=w938:refnum<class "NI-DAQ.lvclass">)  [unwired: 4 in]
          n319 = Replace Array Subset(array=w922, new element=-16.0 ("t"), index=2) -> (w944:dbl[])
          n320 = for {
            N: w941 -> [_]
            tunnel: w923 -> [w979]
            tunnel: w944 -> [w978]
            tunnel: w939 -> [w977]
            tunnel: [w976] -> w950
            tunnel: w938 -> [w975]
            tunnel: [w974] -> w936
            tunnel: [w973] -> w943
            tunnel: w929 -> [w970]
            tunnel: w928 -> [w967]
            tunnel: w924 -> [w969] mode=indexing
            tunnel: w920 -> [w968] mode=indexing
            tunnel: w919 -> [w966]
            tunnel: [w964] -> w915 mode=concatenating
            n321 = flat-sequence {
              tunnel: [w1002] -> w980
              tunnel: w979 -> [w1001]
              tunnel: w978 -> [w1000]
              tunnel: w977 -> [w998]
              tunnel: w975 -> [w992]
              tunnel: [w997] -> w972
              tunnel: [w985] -> w971
              tunnel: w970 -> [w984]
              tunnel: w967 -> [w995]
              tunnel: [w986] -> _
              tunnel: w966 -> [w986]
              tunnel: [w986] -> w965
              tunnel: w980 -> [w1028]
              tunnel: [w1037] -> w976
              tunnel: [w1036] -> _
              tunnel: [w1032] -> w974
              tunnel: [w1009] -> w973
              tunnel: w972 -> [w1034]
              tunnel: w971 -> [w1030]
              tunnel: w969 -> [w1031]
              tunnel: w968 -> [_]
              tunnel: w967 -> [w1010]
              tunnel: w965 -> [_]
              tunnel: [w1003] -> w964
              frame #0 {
                w990 = FALSE ("Write Value")
                w996 = TRUE ("Write Value")
                w983 = 1 ("Write")
                # "pickup module"
                # "release module"
                # "pickup sample from tray"
                n322 = Add(x=w995, y=w1000) -> (x+y=w999:dbl[])
                n323 = call "XYZTheta-2Zspeed Go.vi"("error in (no error)"=w998, "XYZTheta In"=w999, "Motion in"=w1001) -> ("error out"=w993:errorcluster, "Motion out"=w1002:refnum<class "Motion.lvclass">)  [unwired: 6 in, 1 out]
                n324 = call "Time Delay"("error in (no error)"=w993) -> ("error out"=w987:errorcluster)  [unwired: 10 in]
                n325 = call "0"("error in (no error)"=w987) -> ("error out"=w988:errorcluster)  [unwired: 9 in, 1 out]
                n326 = call "WriteReadWait.vi"("Read Value"=w990, "Write Value"=w990, "error in (no error)"=w988, "Read"=w984, "Write"=w984, "I-O in"=w992) -> ("error out"=w989:errorcluster, "I-O out"=w991:refnum<class "NI-DAQ.lvclass">)  [unwired: 4 in]
                n327 = call "Time Delay3"("error in (no error)"=w989) -> ("error out"=w994:errorcluster)  [unwired: 10 in]
                n328 = call "WriteReadWait.vi"("Read Value"=w996, "Write Value"=w996, "error in (no error)"=w994, "Read"=w983, "Write"=w983, "I-O in"=w991) -> ("error out"=w982:errorcluster, "I-O out"=w997:refnum<class "NI-DAQ.lvclass">)  [unwired: 4 in]
                n329 = call "release"("error in (no error)"=w982) -> ("error out"=w981:errorcluster)  [unwired: 9 in, 1 out]
                n330 = call "Delay5"("error in (no error)"=w981) -> ("error out"=w985:errorcluster)  [unwired: 10 in]
              }
              frame #1 {
                w1033 = 1 ("Write")
                w1035 = FALSE ("Write Value")
                # "7mins"
                # "lift for chip/sensor thickness"
                # "place sample on HDI"
                n331 = Add(x=w1031, y=dbl[] [0.0, 0.0, -16.0, 0.0]) -> (x+y=w1026:dbl[])
                n332 = call-dynamic "Get Current Position.vi"("Motion in"=w1028) -> ("XYZTheta Out"=w1024:dbl[], "Motion out"=w1027:refnum<class "Motion.lvclass">)  [unwired: 8 in, 1 out]
                "gantry position test" <- w1024
                n333 = Array Subset(array=w1010, index=0, length=2) -> (w1013:dbl[])
                n334 = Build Array (concatenate)(w1013, 0.0 ("element"), 0.0 ("element")) -> (w1012:dbl[])
                n335 = Subtract(x=w1026, y=w1012) -> (x-y=w1025:dbl[])
                "displacement" <- w1025
                n336 = Array Subset(array=w1024, index=0, length=2) -> (w1019:dbl[])
                n337 = Build Array (concatenate)(w1019, 0.0 ("element"), 0.0 ("element")) -> (w1018:dbl[])
                n338 = Add(x=w1018, y=w1025) -> (x+y=w1007:dbl[])
                n339 = Add(x="offset", y=w1007) -> (x+y=w1003:dbl[])
                "gantry target position" <- w1003
                n340 = call "XYZTheta-2Zspeed Go.vi"("error in (no error)"=w1030, "XYZTheta In"=w1003, "Motion in"=w1027) -> ("error out"=w1029:errorcluster, "XYZTheta Out"=w1036:dbl[], "Motion out"=w1037:refnum<class "Motion.lvclass">)  [unwired: 6 in]
                n341 = call "1"("error in (no error)"=w1029) -> ("error out"=w1006:errorcluster)  [unwired: 9 in, 1 out]
                n342 = call "WriteReadWait.vi"("Read Value"=w1035, "Write Value"=w1035, "error in (no error)"=w1006, "Read"=w1033, "Write"=w1033, "I-O in"=w1034) -> ("error out"=w1005:errorcluster, "I-O out"=w1032:refnum<class "NI-DAQ.lvclass">)  [unwired: 4 in]
                n343 = call "Time Delay6"("error in (no error)"=w1005) -> ("error out"=w1004:errorcluster)  [unwired: 10 in]
                n344 = call "Time Delay4"("error in (no error)"=w1004) -> ("error out"=w1009:errorcluster)  [unwired: 10 in]
              }
            }
          }
          n345 = case shown="True" w918 {
            tunnel: [dbl[] [346.77, 628.513, 53.0078, 0.0] w963] -> w917
            tunnel: w916 -> [_ w963]
            tunnel: w915 -> [w957 w961]
            frame False {
              # "north side"
              n346 = call-poly <vilib>:"Write Delimited Spreadsheet.vi"("file path (dialog if empty)"=path "D:/INTT/V1/Assembly Data/ladder assembly/northtool.txt" ("file path (dialog if empty) 4"), "format (%.3f)"="%.10f", "1D data"=w957) -> ()  [unwired: 11 in, 2 out]
            }
            frame True {
              # "south side"
              n347 = call-poly <vilib>:"Write Delimited Spreadsheet.vi"("file path (dialog if empty)"=path "D:/INTT/V1/Assembly Data/ladder assembly/southtool.txt" ("file path (dialog if empty) 4"), "format (%.3f)"="%.10f", "1D data"=w961) -> ()  [unwired: 11 in, 2 out]
            }
          }
          n348 = call "XYZTheta-2Zspeed Go.vi"("error in (no error)"=w943, "XYZTheta In"=w917, "Motion in"=w950) -> ("error out"=w932:errorcluster, "Motion out"=w954:refnum<class "Motion.lvclass">)  [unwired: 6 in, 1 out]
          n349 = call "Time Delay9"("error in (no error)"=w932) -> ("error out"=w914:errorcluster)  [unwired: 10 in]
          n350 = call "?"("error in (no error)"=w914) -> ("error out"=w913:errorcluster)  [unwired: 9 in, 1 out]
          n351 = call-dynamic "Digital Write 1 Channel.vi"("DAQ Module"=0, "error constant"=w913, "Value"=FALSE, "Channel"=0, "NI-DAQ.lvclass"=w936) -> ("error IO"=w933:errorcluster, "NI-DAQ.lvclass 2"=w935:refnum<class "NI-DAQ.lvclass">)  [unwired: 5 in]
          n352 = call "Time Delay10"("error in (no error)"=w933) -> ("error out"=w951:errorcluster)  [unwired: 10 in]
          n353 = call-dynamic "Z Go.vi"("error in (no error)"=w951, "Speed"=10.0, "Position"=0.0 ("new element/subarray"), "Motion in"=w954) -> ("Motion out"=w947:refnum<class "Motion.lvclass">)  [unwired: 6 in, 1 out]
        }
      }
      event "GOTO": Value Change {
        (unwired) "GOING to a position" ("String")
        n354 = event-data() -> ()  [unwired: 1 in, 6 out]
        n355 = call "XYZTheta Go.vi"("XYZTheta In"="Parking position", "Motion in"=w1075) -> ("Motion out"=w1073:refnum<class "Motion.lvclass">)  [unwired: 7 in, 2 out]
      }
      event "READ Position": Value Change {
        n356 = event-data() -> ()  [unwired: 1 in, 6 out]
        n357 = call-dynamic "Get Current Position.vi"("Motion in"=w1095) -> ("XYZTheta Out"=→"Gantry current position":dbl[], "Motion out"=w1094:refnum<class "Motion.lvclass">)  [unwired: 8 in, 1 out]
      }
      event "HDI vacuum": Value Change {
        n358 = event-data() -> ()  [unwired: 1 in, 6 out]
        n359 = call "WriteReadWait.vi"("Read Value"="vacuum", "Write Value"="vacuum", "Read"=w1108, "Write"=w1108, "I-O in"=w1111) -> ("error out"=w1109:errorcluster, "I-O out"=w1098:refnum<class "NI-DAQ.lvclass">)  [unwired: 5 in]
        n360 = call "Time Delay2"("error in (no error)"=w1109) -> ()  [unwired: 10 in, 1 out]
      }
      event Timeout {
        n361 = event-data() -> ()  [unwired: 1 in, 3 out]
        n362 = call-dynamic "Digital Read 1 Channel.vi"("Read"=w1124, "NI-DAQ in"=w1125) -> ("Value"=→"Status":bool, "NI-DAQ out"=w1123:refnum<class "NI-DAQ.lvclass">)  [unwired: 7 in, 1 out]
      }
    }
    "Measured HDI size" <- w31
    "MPT positions on stave" <- w32
    "Stave mark" <- w30
    "measured HDI top-left position" <- w27
    n363 = feedback-in #1(w31) -> ()
    n364 = feedback-in #2(w30) -> ()
    n365 = feedback-in #3(w27) -> ()
    n366 = feedback-in #4(w16) -> ()
    n367 = feedback-in #5(w42) -> ()
    n368 = feedback-in #6(w39) -> ()
    n369 = feedback-in #7(w47) -> ()
    n370 = feedback-in #8(w32) -> ()
    n371 = feedback-in #9(w48) -> ()
    n372 = feedback-in #10(w11) -> ()
    "# of tasks excuted" <- w44
  }
  n373 = call-dynamic "Disconnect.vi"("Controller in"=w5) -> ()  [unwired: 9 in, 1 out]
  n374 = call-dynamic "Disconnect.vi"("I-O in"=w2) -> ()  [unwired: 9 in, 1 out]
